vi "SynthNV_3_0a.vi"() -> ()   [LabVIEW 2013]
uses:
  <vilib>/Utility/error.llb/DialogType.ctl
  SynthNVsubroutines/instr.lib/lvserial/lvserial.lvlib
  <vilib>/Utility/file.llb/Read Delimited Spreadsheet (DBL).vi
panel:
  out "Power (dBm)":dbl format="%#_4g"
  out "caldata":dbl[][](array[numeric]) format="%0.3f"
  out "COM Error":bool
  out "Device Under Control":string
  in  "Boolean":bool
  in  "Serial Port Select":refnum<visa-resource-name>="COM3"
  in  "Load":bool
  out "Lock":bool
  in  "RF HP":bool=TRUE
  in  "RF On":bool=TRUE
  in  "Dial Tab":enum32{"VFO Dial", "Touch Pad"}(tab)
  in  "Frequency Adjust":i8(knob)=1 scale=1.0..20.0
  in  "Knob Step Size":i32(ring)=3 items=["1KHz", "10KHz", "100KHz", "1MHz", "10MHz", "100MHz", "1GHz"]
  out "Freq (MHz) 3":dbl format="%#_7g"
  in  "KeyPad":T1
  out "KeyPad Out":dbl format="%7_7g"
  in  "Attenuator (dB)":dbl(slide)=-31.5 min=-31.5 max=0.0 step=0.5
  in  "stop":bool
  in  "Tab Control":T2(tab)
  in  "RF  FREQUENCY MHz":dbl=1000.0 min=34.375 max=4400.0 step=1.0 format="%_7g"
  in  "Enter":bool caption="1"
  out "PWR Level":bool
  out "Waveform Chart":dbl(graph)
  out "RF Detector Pwr dBm":dbl=-67.9609375 format="%_5g"
  in  "Read Power":bool
  in  "VREF":dbl=2.52 format="%#_7g"
  in  "POFFSET":dbl=97.0 format="%#_7g"
  in  "Send\nCal":bool
  out "Number\nof Points":dbl format="%#.6g"
  in  "Stop Frequency":dbl=4000.0 min=34.0 max=4400.0 step=0.001 format="%7_7g"
  in  "Step Time (mS)":dbl=0.55 min=0.25 max=10000.0 step=1.0 format="%_8g"
  in  "Step Size MHz":dbl=50.0 min=0.001 max=4200.0 step=1.0 format="%#_7f"
  in  "Enter SZ":bool caption="1"
  in  "Enter Start":bool caption="1"
  in  "Enter Stop":bool caption="1"
  in  "Enter ST":bool caption="1"
  in  "Start Frequency":dbl=50.0 min=34.0 max=4400.0 step=0.001 format="%7_7g"
  in  "Sweep\nOnce":bool
  in  "Sweep\nContinuously":bool
  in  "Mod Tab":enum32{"PULSE Amplitude", "AM"}(tab)
  in  "Mod Style":bool
  in  "PULNUM":bool caption="1"
  in  "PULOFF":bool caption="1"
  in  "PULON":bool caption="1"
  in  "Send Pulse Burst":bool
  out "Duration (uS)":dbl
  in  "Continuous PM":bool
  in  "# of Pulses":u16=100 min=1 step=1 format="%#.5f"
  in  "Off Time (uS)":u16=10 min=1 max=16000 step=1 format="%#.5f"
  in  "On Time (uS)":u16=1 min=1 max=16000 step=1 format="%#.5f"
  in  "AMAMP":bool caption="1"
  in  "AMPWR":bool caption="1"
  in  "AMCYC":bool caption="1"
  in  "AMFREQ":bool caption="1"
  in  "AM Freq (Hz)":dbl=1000.0 min=2.0 max=500000.0 step=10.0 format="%#.6f"
  out "Actual Freq (Hz)":dbl
  out "Duration (ms)":dbl
  in  "Send AM Burst":bool
  in  "# of Cycles":u16=100 min=1 step=1 format="%#.5f"
  in  "Offset":u8 max=62 step=1
  in  "Amplitude (%)":u8=100 min=1 max=100 step=1
  in  "Continuous AM":bool
  in  "Wave Shape":u8(ring) items=["Sine", "Ramp", "Triangle"]
  in  "LUTsize":u8=32 min=2 step=1
  in  "Read Settings\nFrom SynthNV":bool
  out "read buffer":string
  in  "Allow changing\nof Power Detector\ncalibration values":bool
  in  "GP Dig Out J8 P3":bool
  in  "Read A/D \non J8 P2":bool
  in  "Read A/D \non J8 P1":bool
  in  "REF":bool=TRUE
  in  "Program\nEEprom":bool
  in  "Read\nFirmware\nVersion":bool
  out "Version":string
  in  "Program\nReference":bool
  in  "Poll for\nPhase Lock":bool
  out "A/D1":string
  out "A/D2":string
  in  "GP Dig Out J8 P5":bool
  in  "Start Network\nAnalyzer":bool
  out "Frac":i32
  out "Modulus":i32=500
  out "INT":i16=2000
  out "RF Divider":i32=4
  out "Allregout":u32[](array[numeric])=[4194309, 10896444, 1203, 97986, 134254497, 65536000] format="%08x"
  out "PFd(MHz)":dbl=2.0
  in  "PllCntrl":T3={"PLL PWR"=3, "MUX out"=4, "Phase"=1, "Low Noise"=TRUE, "REF X2"=FALSE, "Mute till LD"=TRUE, "Icp"=15, "Band Sel Div"=16, "REF Divide"=5, "Reference(MHz)"=10.0} {"Icp" scale=0.0..15.0; "MUX out" items=["3-State", "GND", "Vcc", "Analog LD", "Digital LD", "REF / R", "RF / N"]; "PLL PWR" scale=0.0..3.0}
  in  "Step Size (MHz)":dbl=0.001
  in  "Send":bool
  in  "Freq (MHz)":dbl=1000.0 format="%_10g"
  in  "Re-init\nDefaults":bool
  # "v3.0a"
  # "Windfreak Technologies"
  # "Thanks to Martin Henz Systemtechnik for the use of lvserial\nwhich avoids the use of NI VISA"
  # "MHz"
  # "Windfreak Technologies, LLC 2018"
  # "Warning: Max RF power into the\ndetector is 10dBm.  The Synthesizer\ncan generate up to +20dBm.  \nPlease use an external attenuator."
  # "Burst"
  # "Peak Amplitude is\nadjusted with slider\nbar on the right"
  # "Adjust Power Slider to get CW\npower back on after a pulse."
  # "Burst"
  # "(Or Update)"
  # "(Watch for LED D3 toggle.)"
  # "This Tab is for experimental purposes only."
  # "RF Freq (MHz)"
  # "REG5"
  # "REG4"
  # "REG3"
  # "REG2"
  # "REG1"
  # "REG0"
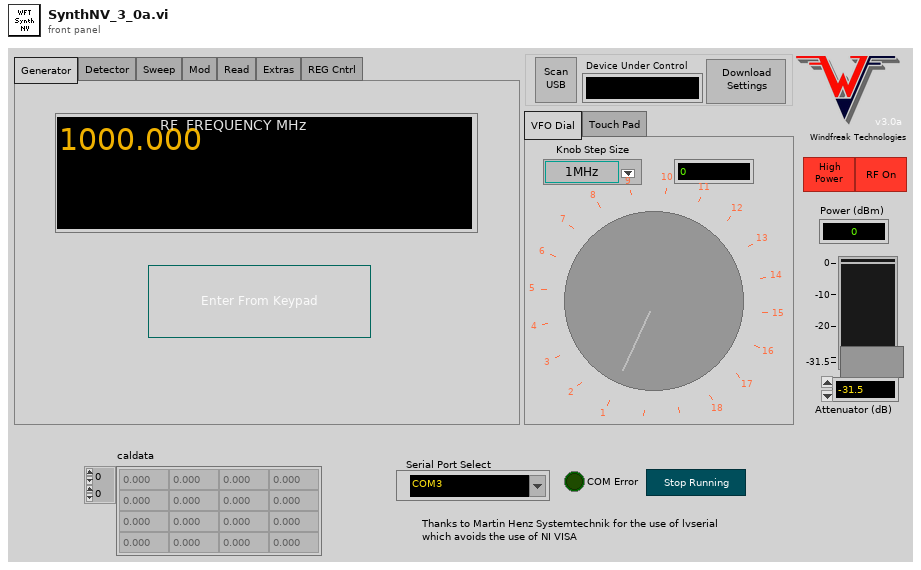
[diagram p1: front panel]
types:
  T1 = cluster{"2":bool, "1":bool, "3":bool, "4":bool, "9":bool, "5":bool, "6":bool, "7":bool, "8":bool, "0":bool, "dp":bool, "Clear":bool}
  T2 = enum32{"Generator", "Detector", "Sweep", "Mod", "Read", "Extras", "REG Cntrl"}
  T3 = cluster{"PLL PWR":i8, "MUX out":u16, "Phase":i16, "Low Noise":bool, "REF X2":bool, "Mute till LD":bool, "Icp":i32, "Band Sel Div":i32, "REF Divide":i16, "Reference(MHz)":dbl}
  T4 = enum8{"Enabled", "Disabled", "Disabled and Grayed Out"}
  T5 = typedef "DialogType.ctl" = u16
  T6 = typedef "LVPoint32TypeDef.ctl" = cluster{"Horizontal":i32, "Vertical":i32}
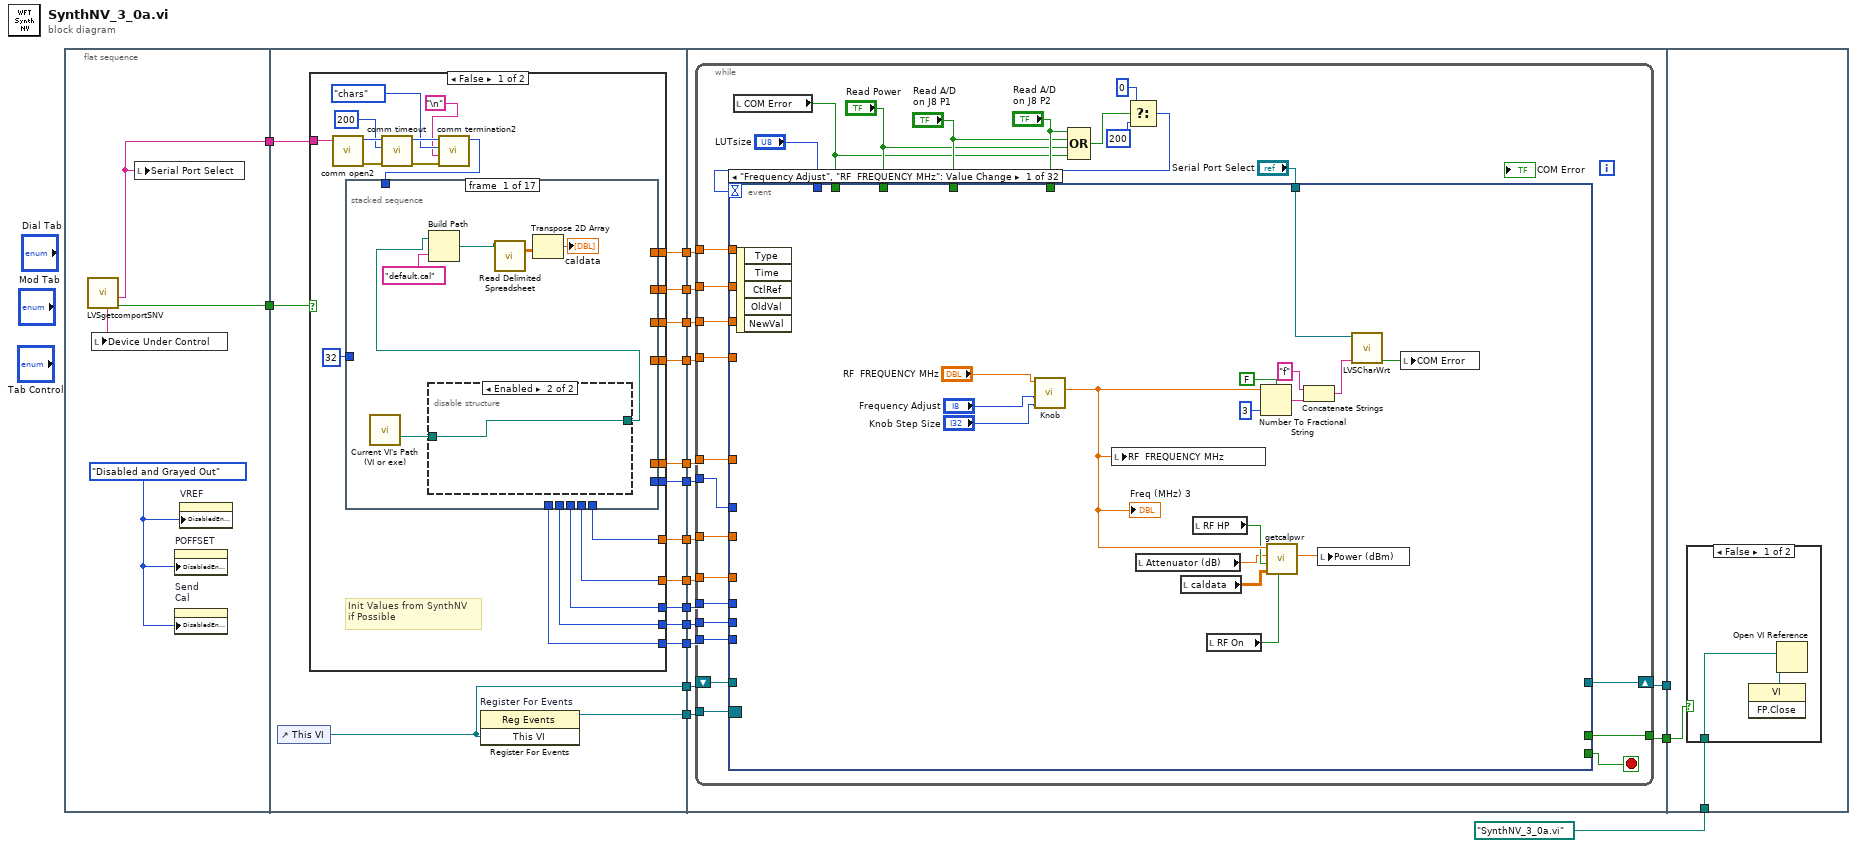
[diagram p0: block diagram]
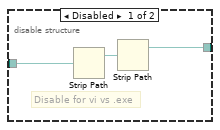
[diagram p2: hidden frame]
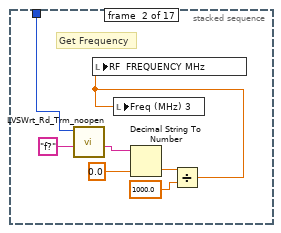
[diagram p3: hidden frame]
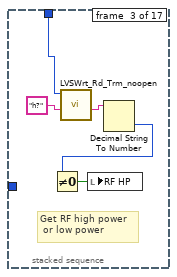
[diagram p4: hidden frame]
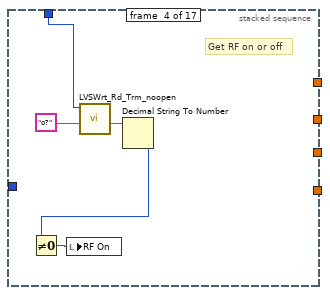
[diagram p5: hidden frame]
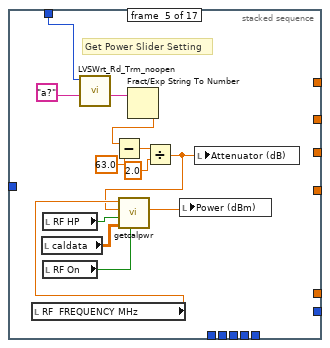
[diagram p6: hidden frame]
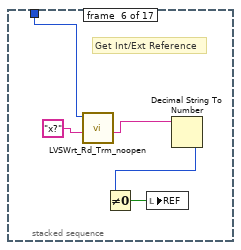
[diagram p7: hidden frame]
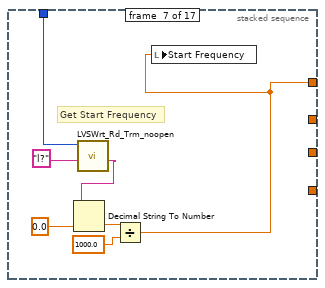
[diagram p8: hidden frame]
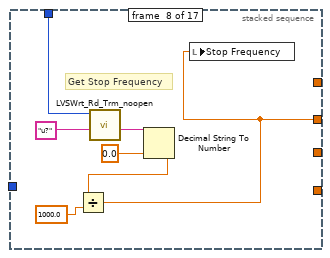
[diagram p9: hidden frame]
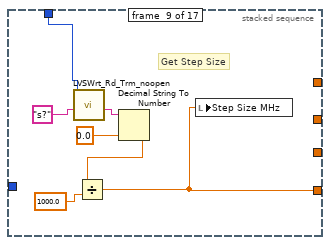
[diagram p10: hidden frame]
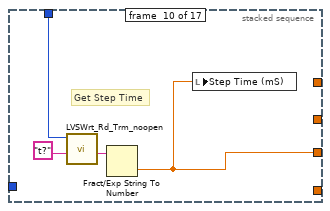
[diagram p11: hidden frame]
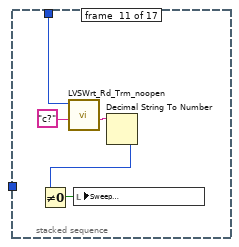
[diagram p12: hidden frame]
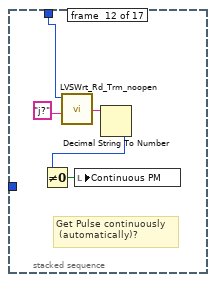
[diagram p13: hidden frame]
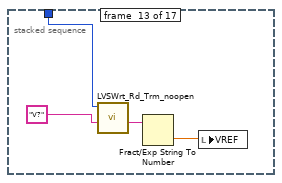
[diagram p14: hidden frame]
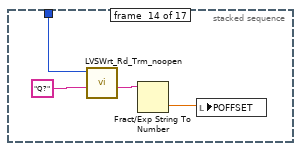
[diagram p15: hidden frame]
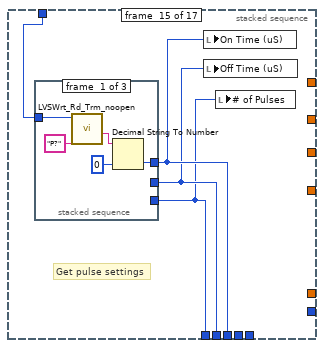
[diagram p16: hidden frame]
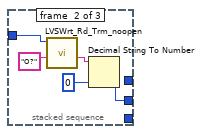
[diagram p17: hidden frame]
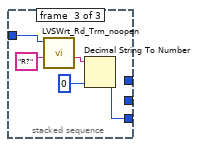
[diagram p18: hidden frame]
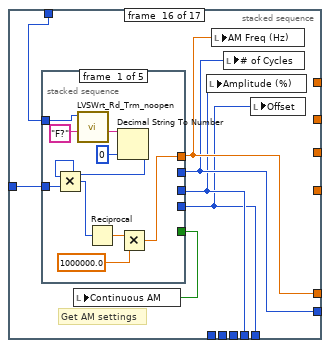
[diagram p19: hidden frame]
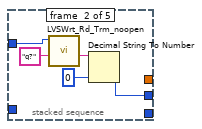
[diagram p20: hidden frame]
diagram:
  n1 = flat-sequence {
    tunnel: [w20] -> w18
    tunnel: [w21] -> w6
    tunnel: w18 -> [w37]
    tunnel: [w36] -> w17
    tunnel: [w35] -> w16
    tunnel: [w34] -> w15
    tunnel: [w33] -> w14
    tunnel: [w32] -> w13
    tunnel: [w31] -> w12
    tunnel: [w30] -> w11
    tunnel: [w29] -> w10
    tunnel: [w28] -> w9
    tunnel: [w27] -> w8
    tunnel: [w26] -> w7
    tunnel: w6 -> [w25]
    tunnel: [w23] -> w5
    tunnel: [w24] -> w4
    tunnel: w17 -> [w236]
    tunnel: w16 -> [w235]
    tunnel: w15 -> [w234]
    tunnel: w14 -> [w233]
    tunnel: w13 -> [w232]
    tunnel: w12 -> [w231]
    tunnel: w11 -> [w230]
    tunnel: w10 -> [w229]
    tunnel: w9 -> [w228]
    tunnel: w8 -> [w227]
    tunnel: w7 -> [w226]
    tunnel: w5 -> [w224]
    tunnel: w4 -> [w225]
    tunnel: [w223] -> w3
    tunnel: [w222] -> w2
    tunnel: w3 -> [_]
    tunnel: w2 -> [w903]
    tunnel: path "SynthNV_3_0a.vi" ("vi path") -> [w902]
    frame #0 {
      w22 = T4."Disabled and Grayed Out" ("Disabled")
      n2 = call "LVSgetcomportSNV.vi"() -> ("No Devices"=w20:bool, "Port"=w21:string, "Device"=w19:string)  [unwired: 9 in]
      n3 = local write "Device Under Control"(w19) -> ()
      n4 = local write "Serial Port Select"(w21) -> ()
      n5 = property on="POFFSET" class="DigNum (strict)"("DisabledEnum"=w22) -> ()  [unwired: 2 in, 2 out]
      n6 = property on="Send\nCal" class="Bool"("DisabledEnum"=w22) -> ()  [unwired: 2 in, 2 out]
      n7 = property on="VREF" class="DigNum (strict)"("DisabledEnum"=w22) -> ()  [unwired: 2 in, 2 out]
    }
    frame #1 {
      n8 = control-ref of="This VI"() -> (w24:refnum<vi>)
      n9 = case shown="False" w37 {
        tunnel: [w58 200.0 ("Start ini")] -> w36
        tunnel: [w57 4000.0 ("upper limit")] -> w35
        tunnel: [w55 u32 5 ("upper limit")] -> w34
        tunnel: [w56 50.0 ("upper limit")] -> w33
        tunnel: [w47 1000.0 ("Amp ini")] -> w32
        tunnel: [w48 u16 100 ("OnT ini")] -> w31
        tunnel: [w50 0.0 ("Amp ini")] -> w30
        tunnel: [w49 31.5 ("Amp ini")] -> w29
        tunnel: [w54 u16 1 ("OnT ini")] -> w28
        tunnel: [w52 u16 15 ("OnT ini")] -> w27
        tunnel: [w53 u16 100 ("OnT ini")] -> w26
        tunnel: w25 -> [w46 _]
        frame False {
          # "Init Values from SynthNV\nif Possible"
          n10 = call "comm open2.vi"("Comm Port Name"=w46) -> ("error out"=w45:errorcluster, "Comm Handle"=w44:u32)  [unwired: 4 in, 1 out]
          n11 = call "comm timeout.vi"("error in (no error)"=w45, "Timeout"=u32 200 ("timeout (10sec)"), "Comm Handle"=w44) -> ("error out"=w42:errorcluster, "dup Comm Handle"=w41:u32)  [unwired: 7 in]
          n12 = call "comm termination2.vi"("error in (no error)"=w42, "termination"="\n", "Termination Mode"=enum16{"none", "chars", "string", "regex"}."chars", "Comm Handle"=w41) -> ("dup Comm Handle"=w38:u32)  [unwired: 6 in, 1 out]
          n13 = stacked-sequence {
            tunnel: u8 32 ("LUTsize") -> [_ _ _ _ _ _ _ _ _ _ _ _ _ _ _ w172 _]
            tunnel: [_ _ _ _ _ _ w107 _ _ _ _ _ _ _ _ _ _] -> w58
            tunnel: [_ _ _ _ _ _ _ w114 _ _ _ _ _ _ _ _ _] -> w57
            tunnel: [_ _ _ _ _ _ _ _ w121 _ _ _ _ _ _ _ _] -> w56
            tunnel: [_ _ _ _ _ _ _ _ _ w128 _ _ _ _ _ _ _] -> w55
            tunnel: [_ _ _ _ _ _ _ _ _ _ _ _ _ _ w150 _ _] -> w54
            tunnel: [_ _ _ _ _ _ _ _ _ _ _ _ _ _ w148 _ _] -> w53
            tunnel: [_ _ _ _ _ _ _ _ _ _ _ _ _ _ w149 _ _] -> w52
            tunnel: [_ _ _ _ _ _ _ _ _ _ _ _ _ _ _ w167 _] -> w50
            tunnel: [_ _ _ _ _ _ _ _ _ _ _ _ _ _ _ w168 _] -> w49
            tunnel: [_ _ _ _ _ _ _ _ _ _ _ _ _ _ _ w169 _] -> w48
            tunnel: [_ _ _ _ _ _ _ _ _ _ _ _ _ _ _ w170 _] -> w47
            tunnel: w38 -> [_ w70 w76 w81 w86 w99 w104 w111 w118 w125 w129 w134 w139 w143 w147 w166 w203]
            frame #0 {
              n14 = call "Current VI's Path (VI or exe).vi"() -> ("VI or executable installation directory"=w60:path)  [unwired: 14 in, 1 out]
              n15 = disable-structure shown="Enabled" {
                disable-tunnel: w60 -> [w67 w68]
                disable-tunnel: [w65 w68] -> w59
                frame Disabled {
                  # "Disable for vi vs .exe"
                  n16 = Strip Path(path=w67) -> (stripped path=w66:path)  [unwired: 1 out]
                  n17 = Strip Path(path=w66) -> (stripped path=w65:path)  [unwired: 1 out]
                }
                frame Enabled {
                }
              }
              n18 = Build Path(base path=w59, name or relative path="default.cal") -> (appended path=w62:path)
              n19 = call-poly <vilib>:"Read Delimited Spreadsheet.vi"("file path (dialog if empty)"=w62) -> ("all rows"=w61:dbl[][])  [unwired: 9 in, 5 out]
              n20 = Transpose 2D Array(2D array=w61) -> (transposed array=→"caldata":dbl[][])
            }
            frame #1 {
              # "Get Frequency"
              n21 = call "LVSWrt_Rd_Trm_noopen.vi"("WriteBuf"="f?" ("write buffer"), "Comm Handle"=w70) -> ("string read"=w69:string)  [unwired: 6 in, 2 out]
              n22 = Decimal String To Number(string=w69, default (0L)=0.0 ("default (0 I32)")) -> (number=w74:dbl)  [unwired: 1 in, 1 out]
              n23 = Divide(x=w74, y=1000.0) -> (x/y=w72:dbl)
              n24 = local write "RF  FREQUENCY MHz"(w72) -> ()
              n25 = local write "Freq (MHz) 3"(w72) -> ()
            }
            frame #2 {
              # "Get RF high power\n or low power"
              n26 = call "LVSWrt_Rd_Trm_noopen.vi"("WriteBuf"="h?" ("write buffer"), "Comm Handle"=w76) -> ("string read"=w78:string)  [unwired: 6 in, 2 out]
              n27 = Decimal String To Number(string=w78) -> (number=w80:i32)  [unwired: 2 in, 1 out]
              n28 = Not Equal To 0?(x=w80) -> (x != 0?=w79:bool)
              n29 = local write "RF HP"(w79) -> ()
            }
            frame #3 {
              # "Get RF on or off"
              n30 = call "LVSWrt_Rd_Trm_noopen.vi"("WriteBuf"="o?" ("write buffer"), "Comm Handle"=w81) -> ("string read"=w83:string)  [unwired: 6 in, 2 out]
              n31 = Decimal String To Number(string=w83) -> (number=w85:i32)  [unwired: 2 in, 1 out]
              n32 = Not Equal To 0?(x=w85) -> (x != 0?=w84:bool)
              n33 = local write "RF On"(w84) -> ()
            }
            frame #4 {
              # "Get Power Slider Setting"
              n34 = local read "RF  FREQUENCY MHz"() -> (w93:dbl)
              n35 = local read "caldata"() -> (w94:dbl[][])
              n36 = local read "RF HP"() -> (w91:bool)
              n37 = local read "RF On"() -> (w90:bool)
              n38 = call "LVSWrt_Rd_Trm_noopen.vi"("WriteBuf"="a?" ("write buffer"), "Comm Handle"=w86) -> ("string read"=w88:string)  [unwired: 6 in, 2 out]
              n39 = Fract/Exp String To Number(string=w88) -> (number=w95:dbl)  [unwired: 3 in, 1 out]
              n40 = Subtract(x=w95, y=63.0) -> (x-y=w96:dbl)
              n41 = Divide(x=w96, y=2.0) -> (x/y=w89:dbl)
              n42 = call "getcalpwr.vi"("RF On"=w90, "caldata"=w94, "RF HP"=w91, "attn"=w89, "freq"=w93) -> ("actual"=w92:dbl)  [unwired: 5 in]
              n43 = local write "Power (dBm)"(w92) -> ()
              n44 = local write "Attenuator (dB)"(w89) -> ()
            }
            frame #5 {
              # "Get Int/Ext Reference"
              n45 = call "LVSWrt_Rd_Trm_noopen.vi"("WriteBuf"="x?" ("write buffer"), "Comm Handle"=w99) -> ("string read"=w100:string)  [unwired: 6 in, 2 out]
              n46 = Decimal String To Number(string=w100) -> (number=w103:i32)  [unwired: 2 in, 1 out]
              n47 = Not Equal To 0?(x=w103) -> (x != 0?=w102:bool)
              n48 = local write "REF"(w102) -> ()
            }
            frame #6 {
              # "Get Start Frequency"
              n49 = call "LVSWrt_Rd_Trm_noopen.vi"("WriteBuf"="l?" ("write buffer"), "Comm Handle"=w104) -> ("string read"=w106:string)  [unwired: 6 in, 2 out]
              n50 = Decimal String To Number(string=w106, default (0L)=0.0 ("default (0 I32)")) -> (number=w109:dbl)  [unwired: 1 in, 1 out]
              n51 = Divide(x=w109, y=1000.0) -> (x/y=w107:dbl)
              n52 = local write "Start Frequency"(w107) -> ()
            }
            frame #7 {
              # "Get Stop Frequency"
              n53 = call "LVSWrt_Rd_Trm_noopen.vi"("WriteBuf"="u?" ("write buffer"), "Comm Handle"=w111) -> ("string read"=w113:string)  [unwired: 6 in, 2 out]
              n54 = Decimal String To Number(string=w113, default (0L)=0.0 ("default (0 I32)")) -> (number=w116:dbl)  [unwired: 1 in, 1 out]
              n55 = Divide(x=w116, y=1000.0) -> (x/y=w114:dbl)
              n56 = local write "Stop Frequency"(w114) -> ()
            }
            frame #8 {
              # "Get Step Size"
              n57 = call "LVSWrt_Rd_Trm_noopen.vi"("WriteBuf"="s?" ("write buffer"), "Comm Handle"=w118) -> ("string read"=w120:string)  [unwired: 6 in, 2 out]
              n58 = Decimal String To Number(string=w120, default (0L)=0.0 ("default (0 I32)")) -> (number=w123:dbl)  [unwired: 1 in, 1 out]
              n59 = Divide(x=w123, y=1000.0) -> (x/y=w121:dbl)
              n60 = local write "Step Size MHz"(w121) -> ()
            }
            frame #9 {
              # "Get Step Time"
              n61 = call "LVSWrt_Rd_Trm_noopen.vi"("WriteBuf"="t?" ("write buffer"), "Comm Handle"=w125) -> ("string read"=w127:string)  [unwired: 6 in, 2 out]
              n62 = Fract/Exp String To Number(string=w127) -> (number=w128:dbl)  [unwired: 3 in, 1 out]
              n63 = local write "Step Time (mS)"(w128) -> ()
            }
            frame #10 {
              n64 = call "LVSWrt_Rd_Trm_noopen.vi"("WriteBuf"="c?" ("write buffer"), "Comm Handle"=w129) -> ("string read"=w131:string)  [unwired: 6 in, 2 out]
              n65 = Decimal String To Number(string=w131) -> (number=w133:i32)  [unwired: 2 in, 1 out]
              n66 = Not Equal To 0?(x=w133) -> (x != 0?=w132:bool)
              n67 = local write "Sweep\nContinuously"(w132) -> ()
            }
            frame #11 {
              # "Get Pulse continuously\n (automatically)?"
              n68 = call "LVSWrt_Rd_Trm_noopen.vi"("WriteBuf"="j?" ("write buffer"), "Comm Handle"=w134) -> ("string read"=w136:string)  [unwired: 6 in, 2 out]
              n69 = Decimal String To Number(string=w136) -> (number=w138:i32)  [unwired: 2 in, 1 out]
              n70 = Not Equal To 0?(x=w138) -> (x != 0?=w137:bool)
              n71 = local write "Continuous PM"(w137) -> ()
            }
            frame #12 {
              n72 = call "LVSWrt_Rd_Trm_noopen.vi"("WriteBuf"="V?" ("write buffer"), "Comm Handle"=w139) -> ("string read"=w141:string)  [unwired: 6 in, 2 out]
              n73 = Fract/Exp String To Number(string=w141) -> (number=w142:dbl)  [unwired: 3 in, 1 out]
              n74 = local write "VREF"(w142) -> ()
            }
            frame #13 {
              n75 = call "LVSWrt_Rd_Trm_noopen.vi"("WriteBuf"="Q?" ("write buffer"), "Comm Handle"=w143) -> ("string read"=w145:string)  [unwired: 6 in, 2 out]
              n76 = Fract/Exp String To Number(string=w145) -> (number=w146:dbl)  [unwired: 3 in, 1 out]
              n77 = local write "POFFSET"(w146) -> ()
            }
            frame #14 {
              # "Get pulse settings"
              n78 = stacked-sequence {
                tunnel: [w154 _ _] -> w150
                tunnel: [_ w160 _] -> w149
                tunnel: [_ _ w165] -> w148
                tunnel: w147 -> [w151 w156 w161]
                frame #0 {
                  n79 = call "LVSWrt_Rd_Trm_noopen.vi"("WriteBuf"="P?" ("write buffer"), "Comm Handle"=w151) -> ("string read"=w153:string)  [unwired: 6 in, 2 out]
                  n80 = Decimal String To Number(string=w153, default (0L)=u16 0 ("default (0 I32)")) -> (number=w154:u16)  [unwired: 1 in, 1 out]
                }
                frame #1 {
                  n81 = call "LVSWrt_Rd_Trm_noopen.vi"("WriteBuf"="O?" ("write buffer"), "Comm Handle"=w156) -> ("string read"=w158:string)  [unwired: 6 in, 2 out]
                  n82 = Decimal String To Number(string=w158, default (0L)=u16 0 ("default (0 I32)")) -> (number=w160:u16)  [unwired: 1 in, 1 out]
                }
                frame #2 {
                  n83 = call "LVSWrt_Rd_Trm_noopen.vi"("WriteBuf"="R?" ("write buffer"), "Comm Handle"=w161) -> ("string read"=w163:string)  [unwired: 6 in, 2 out]
                  n84 = Decimal String To Number(string=w163, default (0L)=u16 0 ("default (0 I32)")) -> (number=w165:u16)  [unwired: 1 in, 1 out]
                }
              }
              n85 = local write "On Time (uS)"(w150) -> ()
              n86 = local write "Off Time (uS)"(w149) -> ()
              n87 = local write "# of Pulses"(w148) -> ()
            }
            frame #15 {
              # "Get AM settings"
              n88 = stacked-sequence {
                tunnel: [_ w187 _ _ _] -> w169
                tunnel: [_ _ w192 _ _] -> w168
                tunnel: [_ _ _ w196 _] -> w167
                tunnel: w172 -> [w181 _ _ _ _]
                tunnel: [w176 _ _ _ _] -> w170
                tunnel: [_ _ _ _ w201] -> w171
                tunnel: w166 -> [w173 w183 w188 w193 w198]
                frame #0 {
                  n89 = call "LVSWrt_Rd_Trm_noopen.vi"("WriteBuf"="F?" ("write buffer"), "Comm Handle"=w173) -> ("string read"=w175:string)  [unwired: 6 in, 2 out]
                  n90 = Decimal String To Number(string=w175, default (0L)=u16 0 ("default (0 I32)")) -> (number=w180:u16)  [unwired: 1 in, 1 out]
                  n91 = Multiply(x=w180, y=w181) -> (x*y=w179:u16)
                  n92 = Reciprocal(x=w179) -> (1/x=w178:dbl)
                  n93 = Multiply(x=w178, y=1000000.0) -> (x*y=w176:dbl)
                }
                frame #1 {
                  n94 = call "LVSWrt_Rd_Trm_noopen.vi"("WriteBuf"="q?" ("write buffer"), "Comm Handle"=w183) -> ("string read"=w185:string)  [unwired: 6 in, 2 out]
                  n95 = Decimal String To Number(string=w185, default (0L)=u16 0 ("default (0 I32)")) -> (number=w187:u16)  [unwired: 1 in, 1 out]
                }
                frame #2 {
                  n96 = call "LVSWrt_Rd_Trm_noopen.vi"("WriteBuf"="%?" ("write buffer"), "Comm Handle"=w188) -> ("string read"=w190:string)  [unwired: 6 in, 2 out]
                  n97 = Decimal String To Number(string=w190, default (0L)=u16 0 ("default (0 I32)")) -> (number=w192:u16)  [unwired: 1 in, 1 out]
                }
                frame #3 {
                  n98 = call "LVSWrt_Rd_Trm_noopen.vi"("WriteBuf"="@?" ("write buffer"), "Comm Handle"=w193) -> ("string read"=w195:string)  [unwired: 6 in, 2 out]
                  n99 = Decimal String To Number(string=w195, default (0L)=u16 0 ("default (0 I32)")) -> (number=w196:u16)  [unwired: 1 in, 1 out]
                }
                frame #4 {
                  # "Cont AM"
                  n100 = call "LVSWrt_Rd_Trm_noopen.vi"("WriteBuf"="A?" ("write buffer"), "Comm Handle"=w198) -> ("string read"=w200:string)  [unwired: 6 in, 2 out]
                  n101 = Decimal String To Number(string=w200) -> (number=w202:i32)  [unwired: 2 in, 1 out]
                  n102 = Not Equal To 0?(x=w202) -> (x != 0?=w201:bool)
                }
              }
              n103 = local write "Continuous AM"(w171) -> ()
              n104 = local write "Amplitude (%)"(w168) -> ()
              n105 = local write "AM Freq (Hz)"(w170) -> ()
              n106 = local write "# of Cycles"(w169) -> ()
              n107 = local write "Offset"(w167) -> ()
            }
            frame #16 {
              w209 = T5 0 items=["no dialog", "OK message", "continue or stop message", "OK message + warnings", "continue/stop + warnings"] ("type of dialog (OK msg:1)")
              # "Close session to port."
              n108 = call "comm close2.vi"("Comm Handle"=w203) -> ("error out"=w204:errorcluster)  [unwired: 6 in]
              n109 = call <vilib>:"Simple Error Handler.vi"("type of dialog (OK msg:1)"=w209, "error in (no error)"=w204) -> ("error?"=w205:bool)  [unwired: 7 out]
              n110 = Equal?(x=w205, y=TRUE) -> (x = y?=w207:bool)
              n111 = case shown="True" w207 {
                tunnel: "Serial Port Error" ("message") -> [_ w210]
                frame False {
                }
                frame True {
                  n112 = Two Button Dialog(message=w210) -> ()  [unwired: 2 in, 1 out]
                }
              }
            }
          }
        }
        frame True {
        }
      }
      n113 = register-events "Register For Events"(w24) -> (reference out=w23:refnum<event-registration>)  [unwired: 2 in, 1 out]
    }
    frame #2 {
      n114 = while {
        tunnel: w235 -> [w262]
        tunnel: w234 -> [w261]
        tunnel: w233 -> [w260]
        tunnel: w236 -> [w259]
        tunnel: w232 -> [w258]
        tunnel: w231 -> [w257]
        tunnel: w230 -> [w252]
        tunnel: w229 -> [w256]
        tunnel: w228 -> [w255]
        tunnel: w227 -> [w254]
        tunnel: w226 -> [w253]
        shift-right: [w247] -> w223
        shift-left: w225 -> [w249]
        tunnel: w224 -> [w248]
        tunnel: [w246] -> w222
        stop <- w250 stop-if-true
        n115 = local read "COM Error"() -> (w240:bool)
        n116 = Compound Arithmetic op=OR("Read A/D \non J8 P2", "Read A/D \non J8 P1", "Read Power", w240) -> (w239:bool)
        n117 = Select(t=0, s=w239, f=200) -> (s? t:f=w238:i32)
        n118 = event shown="[0] \"Frequency Adjust\", \"RF  FREQUENCY MHz\": Value Change" {
          selector: w248 -> [_ _ _ _ _ _ _ _ _ _ _ _ _ _ _ _ _ _ _ _ _ _ _ _ _ _ _ _ _ _ _ _]
          dyn-events: _ -> [_ _ _ _ _ _ _ _ _ _ _ _ _ _ _ _ _ _ _ _ _ _ _ _ _ _ _ _ _ _ _ _]
          timeout: w238 -> [_ _ _ _ _ _ _ _ _ _ _ _ _ _ _ _ _ _ _ _ _ _ _ _ _ _ _ _ _ _ _ _]
          tunnel: w262 -> [_ w312 _ _ _ _ _ _ _ _ _ _ _ _ _ _ _ _ _ _ _ _ _ _ _ _ _ _ _ _ _ _]
          tunnel: w261 -> [_ w311 _ _ _ _ _ _ _ _ _ _ _ _ _ _ _ _ _ _ _ _ _ _ _ _ _ _ _ _ _ _]
          tunnel: w260 -> [_ w310 _ _ _ _ _ _ _ _ _ _ _ _ _ _ _ _ _ _ _ _ _ _ _ _ _ _ _ _ _ _]
          tunnel: w259 -> [_ w309 _ _ _ _ _ _ _ _ _ _ _ _ _ _ _ _ _ _ _ _ _ _ _ _ _ _ _ _ _ _]
          tunnel: w258 -> [_ w288 _ _ _ _ _ _ _ _ _ _ _ _ _ _ _ _ _ _ _ _ _ _ _ _ _ _ _ _ _ _]
          tunnel: w257 -> [_ w287 _ _ _ _ _ _ _ _ _ _ _ _ _ _ _ _ _ _ _ _ _ _ _ _ _ _ _ _ _ _]
          tunnel: w256 -> [_ w286 _ _ _ _ _ _ _ _ _ _ _ _ _ _ _ _ _ _ _ _ _ _ _ _ _ _ _ _ _ _]
          tunnel: w255 -> [_ w279 _ _ _ _ _ _ _ _ _ _ _ _ _ _ _ _ _ _ _ _ _ _ _ _ _ _ _ _ _ _]
          tunnel: w254 -> [_ w280 _ _ _ _ _ _ _ _ _ _ _ _ _ _ _ _ _ _ _ _ _ _ _ _ _ _ _ _ _ _]
          tunnel: w253 -> [_ w285 _ _ _ _ _ _ _ _ _ _ _ _ _ _ _ _ _ _ _ _ _ _ _ _ _ _ _ _ _ _]
          tunnel: w252 -> [_ w282 _ _ _ _ _ _ _ _ _ _ _ _ _ _ _ _ _ _ _ _ _ _ _ _ _ _ _ _ _ _]
          tunnel: "Serial Port Select" -> [w265 _ w324 w341 w368 w404 w416 _ w430 w433 _ w444 w455 w458 w468 w471 w478 w487 w502 _ w578 w602 w610 w617 w622 w624 w639 w646 w664 _ _ w861]
          tunnel: [_ _ _ _ _ _ _ "stop" _ _ _ _ _ _ _ _ _ _ _ _ _ _ _ _ _ _ _ _ _ _ w855 _] -> w250
          tunnel: w249 -> [_ _ _ _ _ _ _ _ _ _ _ _ _ _ _ _ _ _ _ _ _ _ _ _ _ _ _ _ _ _ w854 _]
          tunnel: [_ _ _ _ _ _ _ _ _ _ _ _ _ _ _ _ _ _ _ _ _ _ _ _ _ _ _ _ _ _ w854 _] -> w247
          tunnel: [_ _ _ _ _ _ _ "stop" _ _ _ _ _ _ _ _ _ _ _ _ _ _ _ _ _ _ _ _ _ _ _ _] -> w246
          tunnel: w240 -> [_ _ _ _ _ _ _ _ _ _ _ _ _ _ _ _ _ _ _ _ _ _ _ _ _ _ _ _ _ _ _ w860]
          tunnel: "Read Power" -> [_ _ _ _ _ _ _ _ _ _ _ _ _ _ _ _ _ _ _ _ _ _ _ _ _ _ _ _ _ _ _ w859]
          tunnel: "Read A/D \non J8 P1" -> [_ _ _ _ _ _ _ _ _ _ _ _ _ _ _ _ _ _ _ _ _ _ _ _ _ _ _ _ _ _ _ w858]
          tunnel: "Read A/D \non J8 P2" -> [_ _ _ _ _ _ _ _ _ _ _ _ _ _ _ _ _ _ _ _ _ _ _ _ _ _ _ _ _ _ _ w857]
          tunnel: "LUTsize" -> [_ _ _ _ _ _ _ _ _ _ _ _ _ _ _ w473 w480 _ _ _ _ _ _ _ _ _ _ _ _ w684 _ _]
          event "Frequency Adjust", "RF  FREQUENCY MHz": Value Change {
            n119 = event-data() -> ()  [unwired: 1 in, 5 out]
            n120 = call "Knob.vi"("Freqin"="RF  FREQUENCY MHz", "Knob"="Frequency Adjust", "Knob Step Size"="Knob Step Size") -> ("Freqout"=w271:dbl)  [unwired: 7 in]
            "Freq (MHz) 3" <- w271
            n121 = local write "RF  FREQUENCY MHz"(w271) -> ()
            n122 = local read "Attenuator (dB)"() -> (w266:dbl)
            n123 = local read "caldata"() -> (w270:dbl[][])
            n124 = local read "RF HP"() -> (w268:bool)
            n125 = local read "RF On"() -> (w267:bool)
            n126 = Number To Fractional String(use system decimal point (T)=FALSE, number=w271, precision (6)=i16 3) -> (F-format string=w275:string)  [unwired: 1 in]
            n127 = call "getcalpwr.vi"("RF On"=w267, "caldata"=w270, "RF HP"=w268, "attn"=w266, "freq"=w271) -> ("actual"=w269:dbl)  [unwired: 5 in]
            n128 = Concatenate Strings("f" ("element"), w275) -> (w263:string)
            n129 = local write "Power (dBm)"(w269) -> ()
            n130 = call "LVSCharWrt.vi"("String In"=w263, "COM Port"=w265) -> ("ComError"=w264:bool)  [unwired: 9 in]
            n131 = local write "COM Error"(w264) -> ()
          }
          event "AMPWR", "AMCYC", "Enter Start", "Enter Stop", "Enter ST", "Enter SZ", "AMAMP", "AMFREQ", "PULNUM", "PULOFF", "PULON": Value Change {
            n132 = event-data() -> ()  [unwired: 1 in, 5 out]
            n133 = local read "KeyPad Out"() -> (w281:dbl)
            n134 = call "PulseModEntry.vi"("OnTimeSet"="PULON", "Keypad In"=w281, "OnT ini"=w279, "OffTimeSet"="PULOFF", "OffT ini"=w280, "PulsesSet"="PULNUM", "Pulses ini"=w285) -> ("OnTime"=w296:u16, "OffTime"=w295:u16, "NumPulses"=w283:u32)  [unwired: 4 in, 2 out]
            n135 = call "AMModEntry.vi"("AMFreqSet"="AMFREQ", "Keypad In"=w281, "AMFreq ini"=w288, "NumCycSet"="AMCYC", "NumCyc ini"=w287, "PkPwrSet"="AMPWR", "PkPwr ini"=w282, "AmpSet"="AMAMP", "Amp ini"=w286) -> ("AM Freq"=w300:dbl, "NumCyc"=w299:u16, "PkPwr"=w298:dbl, "Amplitude"=w297:dbl)  [unwired: 2 in, 1 out]
            n136 = call "SweepDataEntry.vi"("Enter Stop"="Enter Stop", "Start ini"=w309, "Enter Start"="Enter Start", "Keypad In"=w281, "Stop ini"=w312, "Enter ST"="Enter ST", "Step ini"=w311, "Enter SZ"="Enter SZ", "SZ ini"=w310) -> ("START FREQUENCY MHz"=w303:dbl, "STOP FREQUENCY MHz"=w304:dbl, "Step Time mS"=w305:dbl, "Step Size MHz"=w306:dbl)  [unwired: 2 in, 1 out]
            n137 = case shown="True" "Enter ST" {
              tunnel: w305 -> [_ w321]
              frame False {
              }
              frame True {
                n138 = local write "Step Time (mS)"(w321) -> ()
              }
            }
            n139 = case shown="True" "Enter SZ" {
              tunnel: w306 -> [_ w320]
              frame False {
              }
              frame True {
                n140 = local write "Step Size MHz"(w320) -> ()
              }
            }
            n141 = case shown="True" "Enter Start" {
              tunnel: w303 -> [_ w323]
              frame False {
              }
              frame True {
                n142 = local write "Start Frequency"(w323) -> ()
              }
            }
            n143 = case shown="True" "Enter Stop" {
              tunnel: w304 -> [_ w322]
              frame False {
              }
              frame True {
                n144 = local write "Stop Frequency"(w322) -> ()
              }
            }
            n145 = case shown="True" "AMAMP" {
              tunnel: w297 -> [_ w316]
              frame False {
              }
              frame True {
                n146 = local write "Amplitude (%)"(w316) -> ()
              }
            }
            n147 = case shown="True" "AMFREQ" {
              tunnel: w300 -> [_ w319]
              frame False {
              }
              frame True {
                n148 = local write "AM Freq (Hz)"(w319) -> ()
              }
            }
            n149 = case shown="True" "AMCYC" {
              tunnel: w299 -> [_ w318]
              frame False {
              }
              frame True {
                n150 = local write "# of Cycles"(w318) -> ()
              }
            }
            n151 = case shown="True" "AMPWR" {
              tunnel: w298 -> [_ w317]
              frame False {
              }
              frame True {
                n152 = local write "Offset"(w317) -> ()
              }
            }
            n153 = case shown="True" "PULON" {
              tunnel: w296 -> [_ w315]
              frame False {
              }
              frame True {
                n154 = local write "On Time (uS)"(w315) -> ()
              }
            }
            n155 = case shown="True" "PULOFF" {
              tunnel: w295 -> [_ w314]
              frame False {
              }
              frame True {
                n156 = local write "Off Time (uS)"(w314) -> ()
              }
            }
            n157 = case shown="True" "PULNUM" {
              tunnel: w283 -> [_ w313]
              frame False {
              }
              frame True {
                n158 = local write "# of Pulses"(w313) -> ()
              }
            }
          }
          event "KeyPad", "Enter": Value Change {
            n159 = event-data() -> ()  [unwired: 1 in, 5 out]
            n160 = call "Keypad.vi"("KeyPad"="KeyPad") -> ("Keypad Out"=w325:dbl)  [unwired: 14 in]
            "KeyPad Out" <- w325
            n161 = case shown="True" "Enter" {
              tunnel: w325 -> [_ w338]
              tunnel: w324 -> [_ w330]
              frame False {
              }
              frame True {
                n162 = In Range and Coerce(upper limit=4500.0, x=w338, lower limit=34.0) -> (coerced(x)=w331:dbl)  [unwired: 1 out]
                n163 = local write "RF  FREQUENCY MHz"(w331) -> ()
                n164 = local write "Freq (MHz) 3"(w331) -> ()
                n165 = Number To Fractional String(use system decimal point (T)=FALSE, number=w331, precision (6)=i16 3) -> (F-format string=w335:string)  [unwired: 1 in]
                n166 = Concatenate Strings("f" ("element"), w335) -> (w329:string)
                n167 = call "LVSCharWrt.vi"("String In"=w329, "COM Port"=w330) -> ("ComError"=w328:bool)  [unwired: 9 in]
                n168 = local write "COM Error"(w328) -> ()
              }
            }
          }
          event "Start Frequency", "Stop Frequency", "Step Time (mS)", "Step Size MHz": Value Change {
            # "Set up processor controlled Sweep\nand computer controlled sweep parameters"
            n169 = event-data() -> ()  [unwired: 1 in, 5 out]
            n170 = Subtract(x="Stop Frequency", y="Start Frequency") -> (x-y=w345:dbl)
            n171 = Divide(x=w345, y="Step Size MHz") -> (x/y=→"Number\nof Points":dbl)
            n172 = Number To Fractional String(use system decimal point (T)=FALSE, number="Step Size MHz", precision (6)=i16 3) -> (F-format string=w353:string)  [unwired: 1 in]
            n173 = Number To Fractional String(use system decimal point (T)=FALSE, number="Step Time (mS)", precision (6)=i16 3) -> (F-format string=w349:string)  [unwired: 1 in]
            n174 = Number To Fractional String(use system decimal point (T)=FALSE, number="Start Frequency", precision (6)=i16 3) -> (F-format string=w365:string)  [unwired: 1 in]
            n175 = Number To Fractional String(use system decimal point (T)=FALSE, number="Stop Frequency", precision (6)=i16 3) -> (F-format string=w357:string)  [unwired: 1 in]
            n176 = Concatenate Strings("d0" ("element"), "r0" ("string"), "l" ("element"), w365, "u" ("element"), w357, "s" ("element"), w353, "t" ("element"), w349) -> (w340:string)
            n177 = call "LVSCharWrt.vi"("String In"=w340, "COM Port"=w341) -> ("ComError"=w339:bool)  [unwired: 9 in]
            n178 = local write "COM Error"(w339) -> ()
          }
          event "On Time (uS)", "Off Time (uS)", "# of Pulses", "Mod Style": Value Change {
            w389 = 500000.0 ("y")
            # "Pulse Modulation"
            n179 = event-data() -> ()  [unwired: 1 in, 5 out]
            n180 = case shown="False" "Mod Style" {
              tunnel: [w392 u8 64] -> w391
              frame False {
                # "(only PDBrf is toggled)"
                # "High Symetry"
                n181 = local read "Attenuator (dB)"() -> (w393:dbl)
                n182 = Multiply(x=w393, y=2.0) -> (x*y=w395:dbl)
                n183 = Add(x=w395, y=63.0) -> (x+y=w397:dbl)
                n184 = To Unsigned Byte Integer(number=w397) -> (unsigned 8bit integer=w392:u8)
              }
              frame True {
                # "PDBrf plus DVGA lines\nare all toggled"
                # "Hi Isolation\nPAM"
              }
            }
            n185 = To Double Precision Float(number="On Time (uS)") -> (double precision float=w376:dbl)
            n186 = To Double Precision Float(number="Off Time (uS)") -> (double precision float=w375:dbl)
            n187 = To Double Precision Float(number="# of Pulses") -> (double precision float=w374:dbl)
            n188 = Add(x=w376, y=w375) -> (x+y=w388:dbl)
            n189 = Number To Decimal String(number="On Time (uS)") -> (decimal integer string=w371:string)  [unwired: 1 in]
            n190 = Number To Decimal String(number="Off Time (uS)") -> (decimal integer string=w372:string)  [unwired: 1 in]
            n191 = Number To Decimal String(number=w391) -> (decimal integer string=w379:string)  [unwired: 1 in]
            n192 = Multiply(x=w388, y=w374) -> (x*y=w384:dbl)
            n193 = Greater?(x=w384, y=w389) -> (0:w386:bool)
            n194 = case shown="True" w386 {
              tunnel: [w399 w401] -> w385
              tunnel: "# of Pulses" -> [w399 _]
              tunnel: w388 -> [_ w402]
              frame False {
              }
              frame True {
                n195 = Divide(x=500000.0 ("y"), y=w402) -> (x/y=w400:dbl)
                n196 = To Unsigned Word Integer(number=w400) -> (unsigned 16bit integer=w401:u16)
              }
            }
            n197 = Number To Decimal String(number=w385) -> (decimal integer string=w373:string)  [unwired: 1 in]
            n198 = Concatenate Strings("P" ("string"), w371, "O" ("string"), w372, "R" ("string"), w373, "M" ("string"), w379) -> (w366:string)
            n199 = call "LVSCharWrt.vi"("String In"=w366, "COM Port"=w368) -> ("ComError"=w367:bool)  [unwired: 9 in]
            n200 = In Range and Coerce(upper limit=w389, x=w384, lower limit=0.0) -> (coerced(x)=→"Duration (uS)":dbl)  [unwired: 1 out]
            n201 = local write "COM Error"(w367) -> ()
          }
          event "Sweep\nContinuously": Value Change {
            # "Sweep Continuously"
            n202 = event-data() -> ()  [unwired: 1 in, 5 out]
            n203 = Boolean To (0,1)(Boolean="Sweep\nContinuously") -> (0, 1=w413:i16)
            n204 = Number To Decimal String(number=w413) -> (decimal integer string=w410:string)  [unwired: 1 in]
            n205 = Concatenate Strings("d" ("element"), "0" ("element"), "c" ("element"), w410, "g" ("element"), w410) -> (w406:string)
            n206 = call "LVSCharWrt.vi"("String In"=w406, "COM Port"=w404) -> ("ComError"=w405:bool)  [unwired: 9 in]
            n207 = local write "COM Error"(w405) -> ()
          }
          event "Send\nCal": Value Change {
            n208 = event-data() -> ()  [unwired: 1 in, 5 out]
            n209 = Number To Fractional String(use system decimal point (T)=FALSE, number="VREF", precision (6)=i16 3) -> (F-format string=w423:string)  [unwired: 1 in]
            n210 = Number To Fractional String(use system decimal point (T)=FALSE, number="POFFSET", precision (6)=i16 3) -> (F-format string=w418:string)  [unwired: 1 in]
            n211 = Concatenate Strings("V" ("element"), w423, "Q" ("string"), w418) -> (w415:string)
            n212 = call "LVSCharWrt.vi"("String In"=w415, "COM Port"=w416) -> ("ComError"=w414:bool)  [unwired: 9 in]
            n213 = local write "COM Error"(w414) -> ()
          }
          event "stop": Value Change {
            n214 = event-data() -> ()  [unwired: 1 in, 5 out]
          }
          event "Read Settings\nFrom SynthNV": Value Change {
            n215 = event-data() -> ()  [unwired: 1 in, 5 out]
            n216 = call "LVSPrtHlp.vi"("VISA resource name"=w430) -> ("error?"=w428:bool, "string read"=→"read buffer":string)  [unwired: 9 in]
            n217 = local write "COM Error"(w428) -> ()
          }
          event "Sweep\nOnce": Value Change {
            # "Sweep Once"
            n218 = event-data() -> ()  [unwired: 1 in, 5 out]
            n219 = Concatenate Strings("d" ("element"), "0" ("element"), "g" ("element"), "1" ("string")) -> (w432:string)
            n220 = local read "Stop Frequency"() -> (w434:dbl)
            n221 = local write "RF  FREQUENCY MHz"(w434) -> ()
            n222 = local write "Freq (MHz) 3"(w434) -> ()
            n223 = call "LVSCharWrt.vi"("String In"=w432, "COM Port"=w433) -> ("ComError"=w431:bool)  [unwired: 9 in]
            n224 = local write "COM Error"(w431) -> ()
          }
          event "Allow changing\nof Power Detector\ncalibration values": Value Change {
            n225 = event-data() -> ()  [unwired: 1 in, 5 out]
            n226 = Select(t=T4."Enabled" ("Disabled"), s="Allow changing\nof Power Detector\ncalibration values", f=T4."Disabled and Grayed Out" ("Disabled")) -> (s? t:f=w440:T4)
            n227 = property on="Send\nCal" class="Bool"("DisabledEnum"=w440) -> ()  [unwired: 2 in, 2 out]
            n228 = property on="VREF" class="DigNum (strict)"("DisabledEnum"=w440) -> ()  [unwired: 2 in, 2 out]
            n229 = property on="POFFSET" class="DigNum (strict)"("DisabledEnum"=w440) -> ()  [unwired: 2 in, 2 out]
          }
          event "Continuous PM": Value Change {
            # "Pulse Continuously"
            n230 = event-data() -> ()  [unwired: 1 in, 5 out]
            n231 = Boolean To (0,1)(Boolean="Continuous PM") -> (0, 1=w449:i16)
            n232 = Select(t=2.0, s="Continuous PM", f=0.0) -> (s? t:f=w452:dbl)
            n233 = Number To Decimal String(number=w449) -> (decimal integer string=w447:string)  [unwired: 1 in]
            n234 = property on="Send Pulse Burst" class="Bool"("DisabledEnum"=w452) -> ()  [unwired: 2 in, 2 out]
            n235 = Concatenate Strings("j" ("element"), w447) -> (w445:string)
            n236 = call "LVSCharWrt.vi"("String In"=w445, "COM Port"=w444) -> ("ComError"=w443:bool)  [unwired: 9 in]
            n237 = local write "COM Error"(w443) -> ()
          }
          event "Send Pulse Burst": Value Change {
            # "Send Pulse Burst"
            n238 = event-data() -> ()  [unwired: 1 in, 5 out]
            n239 = call "LVSCharWrt.vi"("String In"="G" ("write buffer"), "COM Port"=w455) -> ("ComError"=w454:bool)  [unwired: 9 in]
            n240 = local write "COM Error"(w454) -> ()
          }
          event "Continuous AM": Value Change {
            n241 = event-data() -> ()  [unwired: 1 in, 5 out]
            n242 = Select(t=2.0, s="Continuous AM", f=0.0) -> (s? t:f=w464:dbl)
            n243 = property on="Send AM Burst" class="Bool"("DisabledEnum"=w464) -> ()  [unwired: 2 in, 2 out]
            n244 = Boolean To (0,1)(Boolean="Continuous AM") -> (0, 1=w461:i16)
            n245 = Number To Decimal String(number=w461) -> (decimal integer string=w459:string)  [unwired: 1 in]
            n246 = Concatenate Strings("A" ("element"), w459) -> (w456:string)
            n247 = call "LVSCharWrt.vi"("String In"=w456, "COM Port"=w458) -> ("ComError"=w457:bool)  [unwired: 9 in]
            n248 = local write "COM Error"(w457) -> ()
          }
          event "Send AM Burst": Value Change {
            n249 = event-data() -> ()  [unwired: 1 in, 5 out]
            n250 = call "LVSCharWrt.vi"("String In"="B" ("write buffer"), "COM Port"=w468) -> ("ComError"=w466:bool)  [unwired: 9 in]
            n251 = local write "COM Error"(w466) -> ()
          }
          event "LUTsize", "Wave Shape": Value Change {
            # "AM"
            # "Setup Lookup Table for AM"
            n252 = event-data() -> ()  [unwired: 1 in, 5 out]
            n253 = call "AMLUTwaveselect.vi"("Wave Shape"="Wave Shape", "LUTsize"=w473) -> ("Array"=w474:u8[])  [unwired: 1 in]
            n254 = Build Array (concatenate)(u8 9 ("element"), w473, w474) -> (w472:u8[])
            n255 = Byte Array To String(unsigned byte array=w472) -> (string=w469:string)
            n256 = call "LVSCharWrt.vi"("String In"=w469, "COM Port"=w471) -> ("ComError"=w470:bool)  [unwired: 9 in]
            n257 = local write "COM Error"(w470) -> ()
          }
          event "AM Freq (Hz)", "# of Cycles", "Amplitude (%)", "Offset": Value Change {
            n258 = event-data() -> ()  [unwired: 1 in, 5 out]
            n259 = call "AMFreqminduration.vi"("Offset"="Offset", "Amplitude (%)"="Amplitude (%)", "Reps"="# of Cycles", "AM Freq (Hz)"="AM Freq (Hz)", "LUT size"=w480) -> ("Duration (ms)"=→"Duration (ms)":dbl, "AMout"=w479:string, "Actual Freq"=→"Actual Freq (Hz)":dbl)  [unwired: 4 in]
            n260 = call "LVSCharWrt.vi"("String In"=w479, "COM Port"=w478) -> ("ComError"=w477:bool)  [unwired: 9 in]
            n261 = local write "COM Error"(w477) -> ()
          }
          event "PllCntrl", "Send", "Freq (MHz)", "Step Size (MHz)": Value Change {
            # "RAW register writes for controlling\nregisters 2,3,5 especially"
            n262 = event-data() -> ()  [unwired: 1 in, 5 out]
            n263 = call "Getsettings.vi"("PllCntrl"="PllCntrl", "Step Size  (MHz)"="Step Size (MHz)", "Freq (MHz)"="Freq (MHz)") -> ("Modulus"=w492:i32, "INT"=w491:i16, "FRAC"=w490:i32, "RF Divider"=w489:i32, "Pfd (MHz)"=→"PFd(MHz)":dbl)  [unwired: 1 in, 2 out]
            "Frac" <- w490
            "Modulus" <- w492
            "INT" <- w491
            "RF Divider" <- w489
            n264 = call "Get Registers.vi"("Out Divider"=w489, "PllCntrl"="PllCntrl", "INT"=w491, "FRAC"=w490, "MOD"=w492) -> ("concatenated string"=w495:string, "Allregout"=→"Allregout":u32[])  [unwired: 13 in]
            n265 = case shown="True" "Send" {
              tunnel: w487 -> [_ w499]
              tunnel: w495 -> [_ w500]
              frame False {
              }
              frame True {
                n266 = call "LVSCharWrt.vi"("String In"=w500, "COM Port"=w499) -> ("ComError"=w501:bool)  [unwired: 9 in]
                n267 = local write "COM Error"(w501) -> ()
              }
            }
          }
          event "Start Network\nAnalyzer": Value Change {
            n268 = event-data() -> ()  [unwired: 1 in, 5 out]
            n269 = stacked-sequence {
              tunnel: w502 -> [w513 _ _ _ w542]
              frame #0 {
                n270 = local read "Attenuator (dB)"() -> (w504:dbl)
                n271 = Multiply(x=w504, y=2.0) -> (x*y=w510:dbl)
                n272 = Add(x=w510, y=63.0) -> (x+y=w512:dbl)
                n273 = To Unsigned Byte Integer(number=w512) -> (unsigned 8bit integer=w507:u8)
                n274 = Number To Decimal String(number=w507) -> (decimal integer string=w503:string)  [unwired: 1 in]
                n275 = Concatenate Strings("A0j0g0" ("string"), "a" ("element"), w503) -> (w505:string)
                n276 = call "LVSCharWrt.vi"("String In"=w505, "COM Port"=w513) -> ()  [unwired: 9 in, 1 out]
              }
              frame #1 {
                w514 = T4."Disabled and Grayed Out" ("Disabled")
                w515 = TRUE
                w516 = FALSE
                n277 = local write "Sweep\nContinuously"(w516) -> ()
                n278 = local write "Read Power"(w516) -> ()
                n279 = local write "Continuous PM"(w516) -> ()
                n280 = local write "Continuous AM"(w516) -> ()
                n281 = property on="Tab Control" class="TabCtl (strict)"("DisabledEnum"=w514) -> ()  [unwired: 2 in, 2 out]
                n282 = property on="Dial Tab" class="TabCtl (strict)"("DisabledEnum"=w514) -> ()  [unwired: 2 in, 2 out]
                n283 = property on="Boolean" class="Bool"("DisabledEnum"=w514) -> ()  [unwired: 2 in, 2 out]
                n284 = property on="Load" class="Bool"("DisabledEnum"=w514) -> ()  [unwired: 2 in, 2 out]
                n285 = property on="RF On" class="Bool (strict)"("DisabledEnum"=w514) -> ()  [unwired: 2 in, 2 out]
                n286 = property on="Attenuator (dB)" class="Slide (strict)"("DisabledEnum"=w514) -> ()  [unwired: 2 in, 2 out]
                n287 = property on="RF HP" class="Bool (strict)"("DisabledEnum"=w514) -> ()  [unwired: 2 in, 2 out]
                n288 = local write "RF HP"(w515) -> ()
                n289 = local write "RF On"(w515) -> ()
              }
              frame #2 {
                n290 = call "SNV_NA_2_0a.vi"() -> ()  [unwired: 12 in]
              }
              frame #3 {
                w517 = T4."Enabled" ("Disabled")
                n291 = property on="Tab Control" class="TabCtl (strict)"("DisabledEnum"=w517) -> ()  [unwired: 2 in, 2 out]
                n292 = property on="Dial Tab" class="TabCtl (strict)"("DisabledEnum"=w517) -> ()  [unwired: 2 in, 2 out]
                n293 = property on="Boolean" class="Bool"("DisabledEnum"=w517) -> ()  [unwired: 2 in, 2 out]
                n294 = property on="Load" class="Bool"("DisabledEnum"=w517) -> ()  [unwired: 2 in, 2 out]
                n295 = property on="RF On" class="Bool (strict)"("DisabledEnum"=w517) -> ()  [unwired: 2 in, 2 out]
                n296 = property on="Attenuator (dB)" class="Slide (strict)"("DisabledEnum"=w517) -> ()  [unwired: 2 in, 2 out]
                n297 = property on="RF HP" class="Bool (strict)"("DisabledEnum"=w517) -> ()  [unwired: 2 in, 2 out]
              }
              frame #4 {
                w531 = i16 3 ("precision (6)")
                w530 = FALSE ("use system decimal point (T)")
                # "reset all since gui uses same variables as NA"
                n298 = local read "Attenuator (dB)"() -> (w536:dbl)
                n299 = local read "Start Frequency"() -> (w529:dbl)
                n300 = local read "Stop Frequency"() -> (w528:dbl)
                n301 = local read "Step Time (mS)"() -> (w527:dbl)
                n302 = local read "Step Size MHz"() -> (w526:dbl)
                n303 = local read "RF  FREQUENCY MHz"() -> (w518:dbl)
                n304 = Multiply(x=w536, y=2.0) -> (x*y=w538:dbl)
                n305 = Add(x=w538, y=63.0) -> (x+y=w539:dbl)
                n306 = To Unsigned Byte Integer(number=w539) -> (unsigned 8bit integer=w537:u8)
                n307 = Number To Fractional String(use system decimal point (T)=FALSE, number=w518, precision (6)=i16 3) -> (F-format string=w547:string)  [unwired: 1 in]
                n308 = Number To Decimal String(number=w537) -> (decimal integer string=w533:string)  [unwired: 1 in]
                n309 = Number To Fractional String(use system decimal point (T)=w530, number=w527, precision (6)=w531) -> (F-format string=w521:string)  [unwired: 1 in]
                n310 = Number To Fractional String(use system decimal point (T)=w530, number=w526, precision (6)=w531) -> (F-format string=w519:string)  [unwired: 1 in]
                n311 = Number To Fractional String(use system decimal point (T)=w530, number=w529, precision (6)=w531) -> (F-format string=w525:string)  [unwired: 1 in]
                n312 = Number To Fractional String(use system decimal point (T)=w530, number=w528, precision (6)=w531) -> (F-format string=w523:string)  [unwired: 1 in]
                n313 = Concatenate Strings("f" ("element"), w547, "a" ("element"), w533, "l" ("element"), w525, "u" ("element"), w523, "t" ("element"), w521, "s" ("element"), w519) -> (w543:string)
                n314 = call "LVSCharWrt.vi"("String In"=w543, "COM Port"=w542) -> ("ComError"=w541:bool)  [unwired: 9 in]
                n315 = Equal?(x=w541, y=TRUE) -> (x = y?=w549:bool)
                n316 = case shown="True" w549 {
                  tunnel: "Serial Port Error" ("message") -> [_ w551]
                  frame False {
                  }
                  frame True {
                    n317 = Two Button Dialog(message=w551) -> ()  [unwired: 2 in, 1 out]
                  }
                }
              }
            }
          }
          event Mouse Wheel {
            n318 = event-data() -> ("Coords"=w556:T6, "Delta"=w553:i32)  [unwired: 1 in, 8 out]
            n319 = Unbundle By Name(w556) -> ("Horizontal"=w554:i32)
            n320 = Less?(x=w554, y=380) -> (x < y?=w552:bool)
            n321 = case shown="True" w552 {
              tunnel: w553 -> [w563 w573]
              frame False {
                n322 = local read "Attenuator (dB)"() -> (w564:dbl)
                n323 = Divide(x=w563, y=2.0) -> (x/y=w562:dbl)
                n324 = Add(x=w564, y=w562) -> (x+y=w560:dbl)
                n325 = In Range and Coerce(upper limit=0.0, x=w560, lower limit=-31.5) -> (coerced(x)=w559:dbl)  [unwired: 1 out]
                n326 = property on="Attenuator (dB)" class="Slide (strict)"("Val(Sgnl)"=w559) -> ()  [unwired: 2 in, 2 out]
              }
              frame True {
                n327 = local read "Frequency Adjust"() -> (w566:i8)
                n328 = Add(x=w566, y=w573) -> (x+y=w570:i32)
                n329 = Greater?(x=w566, y=i8 19) -> (0:w571:bool)
                n330 = Less?(x=w566, y=i8 1) -> (x < y?=w567:bool)
                n331 = case shown="True" w571 {
                  tunnel: w570 -> [w576 _]
                  tunnel: [w576 i8 1 ("Freqkn")] -> w569
                  frame False {
                  }
                  frame True {
                  }
                }
                n332 = case shown="True" w567 {
                  tunnel: w569 -> [w574 _]
                  tunnel: [w574 i8 19 ("Freqkn")] -> w565
                  frame False {
                  }
                  frame True {
                  }
                }
                n333 = property on="Frequency Adjust" class="Knob (strict)"("Val(Sgnl)"=w565) -> ()  [unwired: 2 in, 2 out]
              }
            }
          }
          event "Re-init\nDefaults": Value Change {
            # "Reinit to defaults"
            n334 = event-data() -> ()  [unwired: 1 in, 5 out]
            n335 = stacked-sequence {
              tunnel: w578 -> [w580 _ w583 _ w600]
              frame #0 {
                # "Set Reference"
                n336 = call "LVSCharWrt.vi"("String In"="*2.0x1" ("write buffer"), "COM Port"=w580) -> ()  [unwired: 9 in, 1 out]
              }
              frame #1 {
                n337 = Wait (ms)(milliseconds to wait=u32 100) -> ()  [unwired: 1 out]
              }
              frame #2 {
                n338 = call "LVSCharWrt.vi"("String In"="H500580005H400A1043CH3000004B3H218015E42H108008FA1H003E80000" ("write buffer"), "COM Port"=w583) -> ("ComError"=w584:bool)  [unwired: 9 in]
                n339 = local write "COM Error"(w584) -> ()
              }
              frame #3 {
                n340 = local write "Step Size (MHz)"(0.001 ("Step Size (MHz)")) -> ()
                n341 = local write "Freq (MHz)"(1000.0 ("Freq (MHz)")) -> ()
                n342 = local read "PllCntrl"() -> (w585:T3)
                n343 = Bundle By Name(cluster=w585, "PLL PWR"=i8 3, "MUX out"=u16 4, "Phase"=i16 1, "Low Noise"=TRUE, "REF X2"=FALSE, "Mute till LD"=TRUE, "Icp"=15, "Band Sel Div"=16, "REF Divide"=i16 5, "Reference(MHz)"=10.0) -> (w598:T3)
                n344 = local write "PllCntrl"(w598) -> ()
              }
              frame #4 {
                w601 = 1000.0 ("RF  FREQUENCY MHz")
                n345 = local write "RF  FREQUENCY MHz"(w601) -> ()
                n346 = local write "Freq (MHz) 3"(w601) -> ()
                n347 = call "LVSCharWrt.vi"("String In"="c0j0G0A0a0o1h1f1000.0e" ("write buffer"), "COM Port"=w600) -> ()  [unwired: 9 in, 1 out]
              }
            }
          }
          event "GP Dig Out J8 P3": Value Change {
            n348 = event-data() -> ()  [unwired: 1 in, 5 out]
            n349 = Boolean To (0,1)(Boolean="GP Dig Out J8 P3") -> (0, 1=w607:i16)
            n350 = Number To Decimal String(number=w607) -> (decimal integer string=w606:string)  [unwired: 1 in]
            n351 = Concatenate Strings("#" ("element"), w606) -> (w604:string)
            n352 = call "LVSCharWrt.vi"("String In"=w604, "COM Port"=w602) -> ("ComError"=w603:bool)  [unwired: 9 in]
            n353 = local write "COM Error"(w603) -> ()
          }
          event "GP Dig Out J8 P5": Value Change {
            n354 = event-data() -> ()  [unwired: 1 in, 5 out]
            n355 = Boolean To (0,1)(Boolean="GP Dig Out J8 P5") -> (0, 1=w613:i16)
            n356 = Number To Decimal String(number=w613) -> (decimal integer string=w612:string)  [unwired: 1 in]
            n357 = Concatenate Strings("$" ("element"), w612) -> (w609:string)
            n358 = call "LVSCharWrt.vi"("String In"=w609, "COM Port"=w610) -> ("ComError"=w611:bool)  [unwired: 9 in]
            n359 = local write "COM Error"(w611) -> ()
          }
          event "Program\nEEprom": Value Change {
            n360 = event-data() -> ()  [unwired: 1 in, 5 out]
            n361 = call "LVSCharWrt.vi"("String In"="e" ("write buffer"), "COM Port"=w617) -> ("ComError"=w618:bool)  [unwired: 9 in]
            n362 = local write "COM Error"(w618) -> ()
          }
          event "Read\nFirmware\nVersion": Value Change {
            n363 = event-data() -> ()  [unwired: 1 in, 5 out]
            n364 = call "LVSWrt_Rd_Trm.vi"("WriteBuf"="v" ("write buffer"), "COM Port"=w622) -> ("ComError"=w619:bool, "string read"=→"Version":string)  [unwired: 8 in]
            n365 = local write "COM Error"(w619) -> ()
          }
          event "Attenuator (dB)": Value Change {
            # "write to VGA"
            n366 = event-data() -> ()  [unwired: 1 in, 5 out]
            n367 = local read "RF  FREQUENCY MHz"() -> (w632:dbl)
            n368 = local read "caldata"() -> (w631:dbl[][])
            n369 = local read "RF HP"() -> (w629:bool)
            n370 = local read "RF On"() -> (w628:bool)
            n371 = call "getcalpwr.vi"("RF On"=w628, "caldata"=w631, "RF HP"=w629, "attn"="Attenuator (dB)", "freq"=w632) -> ("actual"=→"Power (dBm)":dbl)  [unwired: 5 in]
            n372 = Multiply(x="Attenuator (dB)", y=2.0) -> (x*y=w636:dbl)
            n373 = Add(x=w636, y=63.0) -> (x+y=w638:dbl)
            n374 = To Unsigned Byte Integer(number=w638) -> (unsigned 8bit integer=w627:u8)
            n375 = Number To Decimal String(number=w627) -> (decimal integer string=w634:string)  [unwired: 1 in]
            n376 = Concatenate Strings("a" ("element"), w634) -> (w625:string)
            n377 = call "LVSCharWrt.vi"("String In"=w625, "COM Port"=w624) -> ("ComError"=w623:bool)  [unwired: 9 in]
            n378 = local write "COM Error"(w623) -> ()
          }
          event "Program\nReference": Value Change {
            n379 = event-data() -> ()  [unwired: 1 in, 5 out]
            n380 = Boolean To (0,1)(Boolean="REF") -> (0, 1=w643:i16)
            n381 = Number To Decimal String(number=w643) -> (decimal integer string=w644:string)  [unwired: 1 in]
            n382 = Concatenate Strings("x" ("write buffer"), w644) -> (w640:string)
            n383 = call "LVSCharWrt.vi"("String In"=w640, "COM Port"=w639) -> ("ComError"=w641:bool)  [unwired: 9 in]
            n384 = local write "COM Error"(w641) -> ()
          }
          event "RF HP": Value Change {
            n385 = event-data() -> ()  [unwired: 1 in, 5 out]
            n386 = local read "RF  FREQUENCY MHz"() -> (w653:dbl)
            n387 = local read "Attenuator (dB)"() -> (w652:dbl)
            n388 = local read "caldata"() -> (w650:dbl[][])
            n389 = local read "RF On"() -> (w651:bool)
            n390 = Boolean To (0,1)(Boolean="RF HP") -> (0, 1=w656:i16)
            n391 = Number To Decimal String(number=w656) -> (decimal integer string=w655:string)  [unwired: 1 in]
            n392 = call "getcalpwr.vi"("RF On"=w651, "caldata"=w650, "RF HP"="RF HP", "attn"=w652, "freq"=w653) -> ("actual"=w649:dbl)  [unwired: 5 in]
            n393 = Concatenate Strings("h" ("element"), w655) -> (w647:string)
            n394 = local write "Power (dBm)"(w649) -> ()
            n395 = call "LVSCharWrt.vi"("String In"=w647, "COM Port"=w646) -> ("ComError"=w648:bool)  [unwired: 9 in]
            n396 = local write "COM Error"(w648) -> ()
          }
          event "RF On": Value Change {
            # "Setting Frequency\nMake sure calibration\nHappens even if Powered down"
            n397 = event-data() -> ()  [unwired: 1 in, 5 out]
            n398 = local read "RF  FREQUENCY MHz"() -> (w662:dbl)
            n399 = local read "Attenuator (dB)"() -> (w661:dbl)
            n400 = local read "caldata"() -> (w659:dbl[][])
            n401 = local read "RF HP"() -> (w660:bool)
            n402 = call "getcalpwr.vi"("RF On"="RF On", "caldata"=w659, "RF HP"=w660, "attn"=w661, "freq"=w662) -> ("actual"=w658:dbl)  [unwired: 5 in]
            n403 = stacked-sequence {
              tunnel: w664 -> [w665 _ w674]
              tunnel: "RF On" -> [w670 _ w673]
              tunnel: w662 -> [_ _ w675]
              frame #0 {
                n404 = Boolean To (0,1)(Boolean=w670) -> (0, 1=w669:i16)
                n405 = Number To Decimal String(number=w669) -> (decimal integer string=w668:string)  [unwired: 1 in]
                n406 = Concatenate Strings("o" ("element"), w668) -> (w667:string)
                n407 = call "LVSCharWrt.vi"("String In"=w667, "COM Port"=w665) -> ("ComError"=w666:bool)  [unwired: 9 in]
                n408 = local write "COM Error"(w666) -> ()
              }
              frame #1 {
                n409 = Wait (ms)(milliseconds to wait=u32 1) -> ()  [unwired: 1 out]
              }
              frame #2 {
                n410 = case shown="True" w673 {
                  tunnel: w675 -> [_ w679]
                  tunnel: w674 -> [_ w676]
                  frame False {
                  }
                  frame True {
                    n411 = Number To Fractional String(use system decimal point (T)=FALSE, number=w679, precision (6)=i16 3) -> (F-format string=w680:string)  [unwired: 1 in]
                    n412 = Concatenate Strings("f" ("element"), w680) -> (w678:string)
                    n413 = call "LVSCharWrt.vi"("String In"=w678, "COM Port"=w676) -> ("ComError"=w677:bool)  [unwired: 9 in]
                    n414 = local write "COM Error"(w677) -> ()
                  }
                }
              }
            }
            n415 = local write "Power (dBm)"(w658) -> ()
          }
          event "Load", "Boolean": Value Change {
            # "Only send one error."
            # "Scan for Devices"
            # "Load settings from SynthNV"
            n416 = event-data() -> ()  [unwired: 1 in, 5 out]
            n417 = local read "COM Error"() -> (w690:bool)
            n418 = feedback #1() -> (w692:bool)  [unwired: 1 in]
            n419 = Equal?(x=w692, y=FALSE) -> (x = y?=w695:bool)
            n420 = feedback-in #1(w690) -> ()
            n421 = Equal?(x=w690, y=TRUE) -> (x = y?=w694:bool)
            n422 = And(x=w694, y=w695) -> (x .and. y?=w696:bool)
            n423 = Or(x=w696, y="Boolean") -> (x .or. y?=w689:bool)
            n424 = case shown="True" w689 {
              tunnel: [FALSE ("y") w701] -> w687
              frame False {
              }
              frame True {
                n425 = call "LVSgetcomportSNV.vi"() -> ("No Devices"=w699:bool, "Port"=w698:string, "Device"=→"Device Under Control":string)  [unwired: 9 in]
                n426 = local write "Serial Port Select"(w698) -> ()
                n427 = Not(x=w699) -> (.not. x?=w701:bool)
              }
            }
            n428 = Or(x="Load", y=w687) -> (x .or. y?=w685:bool)
            n429 = case shown="True" w685 {
              tunnel: w684 -> [_ w703]
              frame False {
              }
              frame True {
                n430 = local read "Serial Port Select"() -> (w704:refnum<visa-resource-name>)
                n431 = call "comm open2.vi"("Comm Port Name"=w704) -> ("error out"=w708:errorcluster, "Comm Handle"=w709:u32)  [unwired: 4 in, 1 out]
                n432 = call "comm timeout.vi"("error in (no error)"=w708, "Timeout"=u32 200 ("timeout (10sec)"), "Comm Handle"=w709) -> ("error out"=w710:errorcluster, "dup Comm Handle"=w711:u32)  [unwired: 7 in]
                n433 = call "comm termination2.vi"("error in (no error)"=w710, "termination"="\n", "Termination Mode"=enum16{"none", "chars", "string", "regex"}."chars", "Comm Handle"=w711) -> ("dup Comm Handle"=w702:u32)  [unwired: 6 in, 1 out]
                n434 = stacked-sequence {
                  tunnel: w703 -> [_ _ _ _ _ _ _ _ _ _ _ _ _ _ w815 _]
                  tunnel: w702 -> [w713 w719 w724 w730 w742 w747 w754 w761 w768 w772 w777 w782 w786 w790 w809 w846]
                  frame #0 {
                    # "Get Frequency"
                    n435 = call "LVSWrt_Rd_Trm_noopen.vi"("WriteBuf"="f?" ("write buffer"), "Comm Handle"=w713) -> ("string read"=w712:string)  [unwired: 6 in, 2 out]
                    n436 = Decimal String To Number(string=w712, default (0L)=0.0 ("default (0 I32)")) -> (number=w717:dbl)  [unwired: 1 in, 1 out]
                    n437 = Divide(x=w717, y=1000.0) -> (x/y=w715:dbl)
                    n438 = local write "RF  FREQUENCY MHz"(w715) -> ()
                    n439 = local write "Freq (MHz) 3"(w715) -> ()
                  }
                  frame #1 {
                    # "Get RF high power\n or low power"
                    n440 = call "LVSWrt_Rd_Trm_noopen.vi"("WriteBuf"="h?" ("write buffer"), "Comm Handle"=w719) -> ("string read"=w721:string)  [unwired: 6 in, 2 out]
                    n441 = Decimal String To Number(string=w721) -> (number=w723:i32)  [unwired: 2 in, 1 out]
                    n442 = Not Equal To 0?(x=w723) -> (x != 0?=w722:bool)
                    n443 = local write "RF HP"(w722) -> ()
                  }
                  frame #2 {
                    # "Get RF on or off"
                    n444 = call "LVSWrt_Rd_Trm_noopen.vi"("WriteBuf"="o?" ("write buffer"), "Comm Handle"=w724) -> ("string read"=w726:string)  [unwired: 6 in, 2 out]
                    n445 = Decimal String To Number(string=w726) -> (number=w728:i32)  [unwired: 2 in, 1 out]
                    n446 = Not Equal To 0?(x=w728) -> (x != 0?=w727:bool)
                    n447 = local write "RF On"(w727) -> ()
                  }
                  frame #3 {
                    # "Get Power Slider Setting"
                    n448 = local read "RF  FREQUENCY MHz"() -> (w737:dbl)
                    n449 = local read "caldata"() -> (w729:dbl[][])
                    n450 = local read "RF HP"() -> (w735:bool)
                    n451 = local read "RF On"() -> (w734:bool)
                    n452 = call "LVSWrt_Rd_Trm_noopen.vi"("WriteBuf"="a?" ("write buffer"), "Comm Handle"=w730) -> ("string read"=w732:string)  [unwired: 6 in, 2 out]
                    n453 = Fract/Exp String To Number(string=w732) -> (number=w738:dbl)  [unwired: 3 in, 1 out]
                    n454 = Subtract(x=w738, y=63.0) -> (x-y=w739:dbl)
                    n455 = Divide(x=w739, y=2.0) -> (x/y=w733:dbl)
                    n456 = call "getcalpwr.vi"("RF On"=w734, "caldata"=w729, "RF HP"=w735, "attn"=w733, "freq"=w737) -> ("actual"=w736:dbl)  [unwired: 5 in]
                    n457 = local write "Power (dBm)"(w736) -> ()
                    n458 = local write "Attenuator (dB)"(w733) -> ()
                  }
                  frame #4 {
                    # "Get Int/Ext Reference"
                    n459 = call "LVSWrt_Rd_Trm_noopen.vi"("WriteBuf"="x?" ("write buffer"), "Comm Handle"=w742) -> ("string read"=w743:string)  [unwired: 6 in, 2 out]
                    n460 = Decimal String To Number(string=w743) -> (number=w746:i32)  [unwired: 2 in, 1 out]
                    n461 = Not Equal To 0?(x=w746) -> (x != 0?=w745:bool)
                    n462 = local write "REF"(w745) -> ()
                  }
                  frame #5 {
                    # "Get Start Frequency"
                    n463 = call "LVSWrt_Rd_Trm_noopen.vi"("WriteBuf"="l?" ("write buffer"), "Comm Handle"=w747) -> ("string read"=w749:string)  [unwired: 6 in, 2 out]
                    n464 = Decimal String To Number(string=w749, default (0L)=0.0 ("default (0 I32)")) -> (number=w752:dbl)  [unwired: 1 in, 1 out]
                    n465 = Divide(x=w752, y=1000.0) -> (x/y=w750:dbl)
                    n466 = local write "Start Frequency"(w750) -> ()
                  }
                  frame #6 {
                    # "Get Stop Frequency"
                    n467 = call "LVSWrt_Rd_Trm_noopen.vi"("WriteBuf"="u?" ("write buffer"), "Comm Handle"=w754) -> ("string read"=w756:string)  [unwired: 6 in, 2 out]
                    n468 = Decimal String To Number(string=w756, default (0L)=0.0 ("default (0 I32)")) -> (number=w759:dbl)  [unwired: 1 in, 1 out]
                    n469 = Divide(x=w759, y=1000.0) -> (x/y=w757:dbl)
                    n470 = local write "Stop Frequency"(w757) -> ()
                  }
                  frame #7 {
                    # "Get Step Size"
                    n471 = call "LVSWrt_Rd_Trm_noopen.vi"("WriteBuf"="s?" ("write buffer"), "Comm Handle"=w761) -> ("string read"=w763:string)  [unwired: 6 in, 2 out]
                    n472 = Decimal String To Number(string=w763, default (0L)=0.0 ("default (0 I32)")) -> (number=w766:dbl)  [unwired: 1 in, 1 out]
                    n473 = Divide(x=w766, y=1000.0) -> (x/y=w764:dbl)
                    n474 = local write "Step Size MHz"(w764) -> ()
                  }
                  frame #8 {
                    # "Get Step Time"
                    n475 = call "LVSWrt_Rd_Trm_noopen.vi"("WriteBuf"="t?" ("write buffer"), "Comm Handle"=w768) -> ("string read"=w770:string)  [unwired: 6 in, 2 out]
                    n476 = Fract/Exp String To Number(string=w770) -> (number=w771:dbl)  [unwired: 3 in, 1 out]
                    n477 = local write "Step Time (mS)"(w771) -> ()
                  }
                  frame #9 {
                    n478 = call "LVSWrt_Rd_Trm_noopen.vi"("WriteBuf"="c?" ("write buffer"), "Comm Handle"=w772) -> ("string read"=w774:string)  [unwired: 6 in, 2 out]
                    n479 = Decimal String To Number(string=w774) -> (number=w776:i32)  [unwired: 2 in, 1 out]
                    n480 = Not Equal To 0?(x=w776) -> (x != 0?=w775:bool)
                    n481 = local write "Sweep\nContinuously"(w775) -> ()
                  }
                  frame #10 {
                    # "Get Pulse continuously\n (automatically)?"
                    n482 = call "LVSWrt_Rd_Trm_noopen.vi"("WriteBuf"="j?" ("write buffer"), "Comm Handle"=w777) -> ("string read"=w779:string)  [unwired: 6 in, 2 out]
                    n483 = Decimal String To Number(string=w779) -> (number=w781:i32)  [unwired: 2 in, 1 out]
                    n484 = Not Equal To 0?(x=w781) -> (x != 0?=w780:bool)
                    n485 = local write "Continuous PM"(w780) -> ()
                  }
                  frame #11 {
                    n486 = call "LVSWrt_Rd_Trm_noopen.vi"("WriteBuf"="V?" ("write buffer"), "Comm Handle"=w782) -> ("string read"=w784:string)  [unwired: 6 in, 2 out]
                    n487 = Fract/Exp String To Number(string=w784) -> (number=w785:dbl)  [unwired: 3 in, 1 out]
                    n488 = local write "VREF"(w785) -> ()
                  }
                  frame #12 {
                    n489 = call "LVSWrt_Rd_Trm_noopen.vi"("WriteBuf"="Q?" ("write buffer"), "Comm Handle"=w786) -> ("string read"=w788:string)  [unwired: 6 in, 2 out]
                    n490 = Fract/Exp String To Number(string=w788) -> (number=w789:dbl)  [unwired: 3 in, 1 out]
                    n491 = local write "POFFSET"(w789) -> ()
                  }
                  frame #13 {
                    # "Get pulse settings"
                    n492 = stacked-sequence {
                      tunnel: [w797 _ _] -> w793
                      tunnel: [_ w803 _] -> w792
                      tunnel: [_ _ w808] -> w791
                      tunnel: w790 -> [w794 w799 w804]
                      frame #0 {
                        n493 = call "LVSWrt_Rd_Trm_noopen.vi"("WriteBuf"="P?" ("write buffer"), "Comm Handle"=w794) -> ("string read"=w796:string)  [unwired: 6 in, 2 out]
                        n494 = Decimal String To Number(string=w796, default (0L)=u16 0 ("default (0 I32)")) -> (number=w797:u16)  [unwired: 1 in, 1 out]
                      }
                      frame #1 {
                        n495 = call "LVSWrt_Rd_Trm_noopen.vi"("WriteBuf"="O?" ("write buffer"), "Comm Handle"=w799) -> ("string read"=w801:string)  [unwired: 6 in, 2 out]
                        n496 = Decimal String To Number(string=w801, default (0L)=u16 0 ("default (0 I32)")) -> (number=w803:u16)  [unwired: 1 in, 1 out]
                      }
                      frame #2 {
                        n497 = call "LVSWrt_Rd_Trm_noopen.vi"("WriteBuf"="R?" ("write buffer"), "Comm Handle"=w804) -> ("string read"=w806:string)  [unwired: 6 in, 2 out]
                        n498 = Decimal String To Number(string=w806, default (0L)=u16 0 ("default (0 I32)")) -> (number=w808:u16)  [unwired: 1 in, 1 out]
                      }
                    }
                    n499 = local write "On Time (uS)"(w793) -> ()
                    n500 = local write "Off Time (uS)"(w792) -> ()
                    n501 = local write "# of Pulses"(w791) -> ()
                  }
                  frame #14 {
                    # "Get AM settings"
                    n502 = stacked-sequence {
                      tunnel: [_ w830 _ _ _] -> w812
                      tunnel: [_ _ w835 _ _] -> w811
                      tunnel: [_ _ _ w839 _] -> w810
                      tunnel: w815 -> [w824 _ _ _ _]
                      tunnel: [w819 _ _ _ _] -> w813
                      tunnel: [_ _ _ _ w844] -> w814
                      tunnel: w809 -> [w816 w826 w831 w836 w841]
                      frame #0 {
                        n503 = call "LVSWrt_Rd_Trm_noopen.vi"("WriteBuf"="F?" ("write buffer"), "Comm Handle"=w816) -> ("string read"=w818:string)  [unwired: 6 in, 2 out]
                        n504 = Decimal String To Number(string=w818, default (0L)=u16 0 ("default (0 I32)")) -> (number=w823:u16)  [unwired: 1 in, 1 out]
                        n505 = Multiply(x=w823, y=w824) -> (x*y=w822:u16)
                        n506 = Reciprocal(x=w822) -> (1/x=w821:dbl)
                        n507 = Multiply(x=w821, y=1000000.0) -> (x*y=w819:dbl)
                      }
                      frame #1 {
                        n508 = call "LVSWrt_Rd_Trm_noopen.vi"("WriteBuf"="q?" ("write buffer"), "Comm Handle"=w826) -> ("string read"=w828:string)  [unwired: 6 in, 2 out]
                        n509 = Decimal String To Number(string=w828, default (0L)=u16 0 ("default (0 I32)")) -> (number=w830:u16)  [unwired: 1 in, 1 out]
                      }
                      frame #2 {
                        n510 = call "LVSWrt_Rd_Trm_noopen.vi"("WriteBuf"="%?" ("write buffer"), "Comm Handle"=w831) -> ("string read"=w833:string)  [unwired: 6 in, 2 out]
                        n511 = Decimal String To Number(string=w833, default (0L)=u16 0 ("default (0 I32)")) -> (number=w835:u16)  [unwired: 1 in, 1 out]
                      }
                      frame #3 {
                        n512 = call "LVSWrt_Rd_Trm_noopen.vi"("WriteBuf"="@?" ("write buffer"), "Comm Handle"=w836) -> ("string read"=w838:string)  [unwired: 6 in, 2 out]
                        n513 = Decimal String To Number(string=w838, default (0L)=u16 0 ("default (0 I32)")) -> (number=w839:u16)  [unwired: 1 in, 1 out]
                      }
                      frame #4 {
                        # "Cont AM"
                        n514 = call "LVSWrt_Rd_Trm_noopen.vi"("WriteBuf"="A?" ("write buffer"), "Comm Handle"=w841) -> ("string read"=w843:string)  [unwired: 6 in, 2 out]
                        n515 = Decimal String To Number(string=w843) -> (number=w845:i32)  [unwired: 2 in, 1 out]
                        n516 = Not Equal To 0?(x=w845) -> (x != 0?=w844:bool)
                      }
                    }
                    n517 = local write "Continuous AM"(w814) -> ()
                    n518 = local write "Amplitude (%)"(w811) -> ()
                    n519 = local write "AM Freq (Hz)"(w813) -> ()
                    n520 = local write "# of Cycles"(w812) -> ()
                    n521 = local write "Offset"(w810) -> ()
                  }
                  frame #15 {
                    w852 = T5 0 items=["no dialog", "OK message", "continue or stop message", "OK message + warnings", "continue/stop + warnings"] ("type of dialog (OK msg:1)")
                    # "Close session to port."
                    n522 = call "comm close2.vi"("Comm Handle"=w846) -> ("error out"=w847:errorcluster)  [unwired: 6 in]
                    n523 = call <vilib>:"Simple Error Handler.vi"("type of dialog (OK msg:1)"=w852, "error in (no error)"=w847) -> ("error?"=w848:bool)  [unwired: 7 out]
                    n524 = Equal?(x=w848, y=TRUE) -> (x = y?=w850:bool)
                    n525 = case shown="True" w850 {
                      tunnel: "Serial Port Error" ("message") -> [_ w853]
                      frame False {
                      }
                      frame True {
                        n526 = Two Button Dialog(message=w853) -> ()  [unwired: 2 in, 1 out]
                      }
                    }
                  }
                }
              }
            }
          }
          event Panel Close? {
            w855 = TRUE ("Discard?")
            n527 = event-data() -> ("VIRef"=w856:refnum<vi>)  [unwired: 1 in]
            n528 = Close Reference(reference=w856) -> ()  [unwired: 1 in, 1 out]
            n529 = event-data("Discard?"=w855) -> ()  [unwired: 1 in, 1 out]
          }
          event Timeout {
            n530 = event-data() -> ()  [unwired: 1 in, 2 out]
            n531 = stacked-sequence {
              tunnel: w861 -> [w863 w874 w891 w897]
              tunnel: w860 -> [_ _ _ _]
              tunnel: w859 -> [w862 _ _ _]
              tunnel: w858 -> [_ _ w890 _]
              tunnel: w857 -> [_ _ _ w896]
              frame #0 {
                # "RF Detector vs Time Routine"
                n532 = case shown="True" w862 {
                  tunnel: w863 -> [_ w868]
                  frame False {
                    n533 = Wait (ms)(milliseconds to wait=u32 10) -> ()  [unwired: 1 out]
                  }
                  frame True {
                    # "Measure Pwr"
                    n534 = call "LVSWrt_Rd_Trm.vi"("WriteBuf"="w" ("write buffer"), "COM Port"=w868) -> ("ComError"=w865:bool, "string read"=w867:string)  [unwired: 8 in]
                    n535 = local write "COM Error"(w865) -> ()
                    n536 = Fract/Exp String To Number(use system decimal point (T)=FALSE, string=w867) -> (number=w871:dbl)  [unwired: 2 in, 1 out]
                    "RF Detector Pwr dBm" <- w871
                    "Waveform Chart" <- w871
                    n537 = Greater?(x=w871, y=10.0) -> (0:→"PWR Level":bool)
                  }
                }
              }
              frame #1 {
                # "Poll every second for Phase Lock"
                n538 = case shown="True" "Poll for\nPhase Lock" {
                  tunnel: w874 -> [_ w881]
                  frame False {
                    n539 = property on="Lock" class="Bool (strict)"("Visible"=FALSE) -> ()  [unwired: 2 in, 2 out]
                  }
                  frame True {
                    n540 = Get Date/Time In Seconds() -> (seconds since 1Jan1904=w877:timestamp)
                    n541 = To Double Precision Float(number=w877) -> (double precision float=w879:dbl)
                    n542 = feedback #2() -> (w878:dbl)  [unwired: 1 in]
                    n543 = Round Toward -Infinity(1:w879) -> (0:w880:dbl)
                    n544 = feedback-in #2(w880) -> ()
                    n545 = Not Equal?(x=w880, y=w878) -> (x != y?=w876:bool)
                    n546 = case shown="True" w876 {
                      tunnel: w881 -> [_ w885]
                      frame False {
                      }
                      frame True {
                        n547 = call "LVSWrt_Rd_Trm.vi"("WriteBuf"="p" ("write buffer"), "COM Port"=w885) -> ("ComError"=w882:bool, "string read"=w883:string)  [unwired: 8 in]
                        n548 = local write "COM Error"(w882) -> ()
                        n549 = Fract/Exp String To Number(string=w883) -> (number=w889:dbl)  [unwired: 3 in, 1 out]
                        n550 = Not Equal?(x=0.0, y=w889) -> (x != y?=→"Lock":bool)
                        n551 = property on="Lock" class="Bool (strict)"("Visible"=TRUE) -> ()  [unwired: 2 in, 2 out]
                      }
                    }
                  }
                }
              }
              frame #2 {
                n552 = case shown="True" w890 {
                  tunnel: w891 -> [_ w895]
                  frame False {
                  }
                  frame True {
                    n553 = call "LVSWrt_Rd_Trm.vi"("WriteBuf"="C1" ("write buffer"), "COM Port"=w895) -> ("ComError"=w892:bool, "string read"=→"A/D1":string)  [unwired: 8 in]
                    n554 = local write "COM Error"(w892) -> ()
                  }
                }
              }
              frame #3 {
                n555 = case shown="True" w896 {
                  tunnel: w897 -> [_ w898]
                  frame False {
                  }
                  frame True {
                    n556 = call "LVSWrt_Rd_Trm.vi"("WriteBuf"="C2" ("write buffer"), "COM Port"=w898) -> ("ComError"=w900:bool, "string read"=→"A/D2":string)  [unwired: 8 in]
                    n557 = local write "COM Error"(w900) -> ()
                  }
                }
              }
            }
          }
        }
      }
    }
    frame #3 {
      n558 = case shown="False" w903 {
        tunnel: w902 -> [w904 _]
        frame False {
          n559 = Open VI Reference(vi path=w904) -> (vi reference=w905:refnum<vi>)  [unwired: 5 in, 1 out]
          n560 = invoke class="VI" method="FP.Close"(reference=w905) -> ()  [unwired: 2 in, 3 out]
        }
        frame True {
        }
      }
    }
  }
